vi "AlliGator FLI Dataset Series Actions.vi"(0 "AlliGator Q Elements":T6[](array[typedef]), 1 "VI in":refnum<vi>, 2 "Script in":bool, 5 "AlliGator IV DVR in":refnum<data-value>, 7 "AlliGator Q Event in":T7=enum."GUI:Idle", 9 "Data":variant, 11 "error in (no error)":errorcluster, 12 "AlliGator Ctrl Refnums":T8) -> (3 "Script out":bool, 4 "Alligator Queue Elements":T6[](array[typedef]), 6 "AlliGator IV DVR out":refnum<data-value>, 10 "[Notebook Message]":T1[](array[typedef]) {"Message Style"."Font Size" min=6.0 step=1.0}, 15 "error out":errorcluster)   [LabVIEW 2021, in "AlliGator Action Engine.lvlib"]
doc: "Processes AlliGator FLI Dataset Series-related actions."
uses:
  AlliGator Action Engine.lvlib
  Internal Variables/AlliGator Internal Variables v2.ctl
  <vilib>/vision/Image Controls.llb/IMAQ Image.ctl
  Internal Variables/AlliGator Gate Image Set.ctl
  Files/AlliGator FLI Dataset Type.ctl
  Files/AlliGator Data Series Type.ctl
  Dual-Channel Datasets/AlliGator Dataset Channel.ctl
  Settings/AlliGator Gate Arithmetic.ctl
  Source Image/AlliGator Displayed Image.ctl
  Image/Named ROI Description.ctl
  Phasor Graph/AlliGator Decay Metadata v3.ctl
  Decay Analysis/Decay Preprocessing/AlliGator Decay Background Subtraction Info.ctl
  Decay Analysis/Decay Preprocessing/AlliGator Baseline Subtraction Method.ctl
  Graphs/XY Graph/XY Graph Plot Shift Parameters.ctl
  Graphs/XY Graph/XY Graph Plot Shift Method.ctl
  Decay Analysis/Decay Preprocessing/AlliGator Decay Extrapolation Parameters.ctl
  Phasor/Calibration Phasor (m, phi).ctl
  Phasor/Phasor Reference Series.ctl
  Phasor/Phasor Calibration Map v2.ctl
  Phasor/Phasor (g, s).ctl
  Phasor Graph/AlliGator Raw Phasor Plot Data v5.ctl
  Phasor/Phasor Standard Deviation Options.ctl
  Phasor Plot/AlliGator Phasor Multi-Harmonic Data.ctl
  Phasor/Phasor Harmonic Data.ctl
  Decay Fit Parameter Map/AlliGator Decay Fit Options & Parameters v4.ctl
  Fits/IRF(X)PSED/Decay Fit Options v4.ctl
  Fits/Decay Convolution/Decay Model.ctl
  Fits/Residual Type.ctl
  Fits/IRF(X)PSED/Fit Weights Type v2.ctl
  Fits/Non-linear Fitting Method v2.ctl
  Fits/Fit Calculation Method.ctl
  Fits/Non-linear Fitting Algorithm.ctl
  Decay Analysis/Decay Fit/AlliGator Decay Fit Parameter Constraints 2.ctl
  Fits/IRF(X)PSED/Decay Fit Parameters In List.ctl
  Fits/IRF(X)PSED/MLE Baseline Offset Type.ctl
  Decay Analysis/Decay Preprocessing/AlliGator Decay Preprocessing Parameters.ctl
  Fits/IRF(X)PSED/Decay Fit Parameters & Derived Quantities List v2.ctl
  Fits/IRF(X)PSED/Decay Fit Result Constraint.ctl
  Decay Fit Parameter Map/AlliGator Parameter Maps Data.ctl
  AlliGator Q Event.ctl
  GUI/AlliGator Ctrl Refnums.ctl
  GUI/AlliGator Other Ctrl Refnums.ctl
  GUI/AlliGator State Indicator.ctl
  GUI/AlliGator Main Window Tabs.ctl
  GUI/AlliGator Phasor Plot Ctrl Refnums.ctl
  GUI/AlliGator Phasor Graph Ctrl Refnums.ctl
  Phasor/Phasor Calibration Type.ctl
  GUI/AlliGator Dataset Ctrl Refnums.ctl
  GUI/AlliGator Registered Events Ctrl Refnums.ctl
  GUI/AlliGator Image Histogram Control Refnums.ctl
  Histograms/Linear Histogram Options.ctl
  Histograms/Histogram Bin Option.ctl
  Histograms/Histogram Bin Position.ctl
  Decay Fit Parameter Map/AlliGator Decay Fit Map Control Refnums.ctl
  Parameter Map/AlliGator Parameter Map Control Refnums.ctl
  AlliGator Q Element.ctl
  Notebook/Notebook Message Object.ctl
  Rich Text Box/Text Formatting.ctl
  Rich Text Box/Text Colors.ctl
  Rich Text Box/Text Style.ctl
  Rich Text Box/Text Alignment.ctl
  Rich Text Box/Text Format List.ctl
  Alligator Elements Order in Action Stack.ctl
  Globals, Variables, Constants/AlliGator Variables List.ctl
  Scripts/AlliGator Series Analysis Type.ctl
  Globals, Variables, Constants/AlliGator Globals.vi
  Variant/Variant to Data/Variant to DBL.vi
  Variant/Variant to Data/Variant to Boolean.vi
  AlliGator Add Action Array to Stack.vi
  GUI/GUI.lvlib
  Accumulated Dataset/AlliGator Accumulated Dataset.lvlib
  Scripts/AlliGator Scripts.lvlib
  Sound/Sound.lvlib
  Decay Analysis/Decay Fit/AlliGator Decay Fit.lvlib
  Internal Variables/AlliGator Internal Variables.lvlib
  Image/Image.lvlib
  Variant/Variant to Data/Variant to Data.lvlib
  Source Image/AlliGator Source Image.lvlib
  Globals, Variables, Constants/AlliGator Globals, Variables & Constants.lvlib
  Notebook/Notebook.lvlib
  Phasor/Phasor.lvlib
  Decay Analysis/Decay Preprocessing/AlliGator Decay Preprocessing.lvlib
  Graphs/XY Graph/XY Graph Add-Ons.lvlib
  Phasor Graph/AlliGator Phasor Graph.lvlib
  Files/AlliGator Files.lvlib
  Phasor Plot/AlliGator Phasor Plot.lvlib
  Fits/Fits.lvlib
  Settings/AlliGator Settings.lvlib
  GUI/AlliGator GUI.lvlib
  Decay Fit Parameter Map/AlliGator Decay Fit Parameter Map.lvlib
  Rich Text Box/Rich Text Box.lvlib
  Dual-Channel Datasets/AlliGator Dual-Channel Datasets.lvlib
  Histograms/Histogram Window.lvlib
  Parameter Map/AlliGator Parameter Map.lvlib
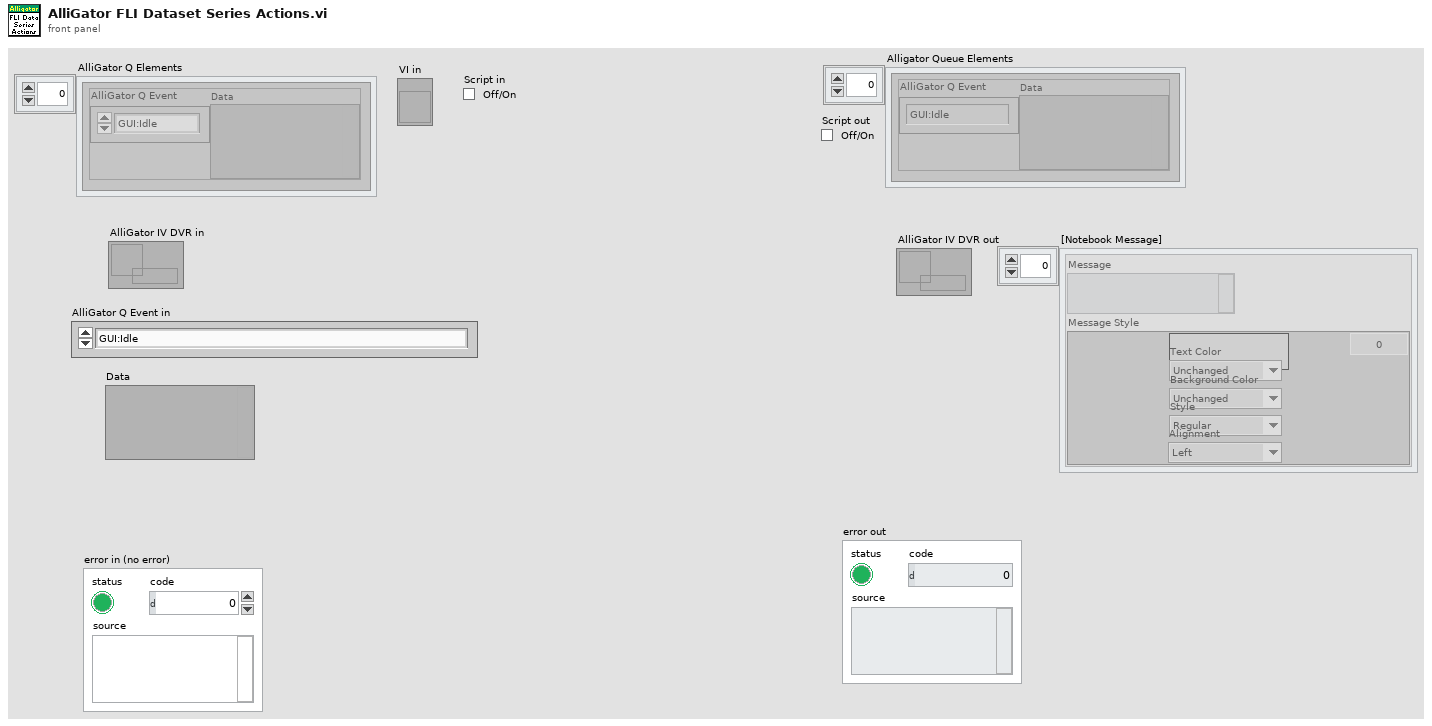
[diagram p1: front panel]
types:
  T1 = typedef "Notebook.lvlib/Notebook Message Object.ctl" = cluster{"Message":string, "Message Style":T2}
  T2 = typedef "Rich Text Box.lvlib/Text Formatting.ctl" = cluster{"Font":string, "Text Color":T3, "Background Color":T3, "Style":T4, "Font Size":dbl, "Alignment":T5}
  T3 = typedef "Rich Text Box.lvlib/Text Colors.ctl" = enum16{"Unchanged", "Black", "Blue", "Cyan", "Maroon", "Gray", "Violet", "Green", "Light Green", "Orange", "Yellow", "Magenta", "Red", "White"}
  T4 = typedef "Rich Text Box.lvlib/Text Style.ctl" = enum16{"Regular", "Bold", "Italic", "Underline", "Strikeout"}
  T5 = typedef "Rich Text Box.lvlib/Text Alignment.ctl" = enum16{"Left", "Right", "Center"}
  T6 = typedef "AlliGator Action Engine.lvlib/AlliGator Q Element.ctl" = cluster{"AlliGator Q Event":T7, "Data":variant}
  T7 = typedef "AlliGator Action Engine.lvlib/AlliGator Q Event.ctl" = enum16{"---- Files ----", "Files:Set Batch Export Files To Save", "Files:Set Dataset Loading & Pre-processing Options", "Files:Check #Frames in Dataset", "Files:Increment Frame Index", "Files:Open Mask Image", "Files:Open White Light Image", "Files:Open Single Dataset", "Files:New Folder of Folders Selected", "Files:Load File (all Types)_Scriptable", "Files:Move Flattened Series to Folders Series", "Files:Select Folder", "Files:Load FLI Dataset", "Files:Load Swiss SPAD 1 Dataset", "Files:Load Swiss SPAD 2 Dataset", "Files:Load .sdt FLI Dataset", "Files:Load .ptu FLI Dataset", "Files:Load .bin FLI Dataset", "Files:Load Single Gate Image Folder", "Files:Load I/m/phi Dataset (deprecated)", "Files:Load Single Image", "Files:Subtract Background File", "Files:Export FLI Dataset", "Files:Load HDF5 FLI Dataset", "Files:Set Destination File Path", "Files:Save Mask Image", "Files:Batch Conversion", "Files:New Folder Selected", "Files:Close FLI Dataset", "Files:Close FLI Dataset Series", "Files:Close White Light Image", "Files:Close Mask Image", "---- FLI Dataset ----", "FLI Dataset:Channel Arithmetic", "FLI Dataset:Export Average Lifetime Map as ASCII", "FLI Dataset:Export User-Defined Quantity Map as ASCII", "FLI Dataset:Python Function FLI Dataset Event", "FLI Dataset:ROI Analysis", "FLI Dataset:Tilted Logistic Square Gated IRF Characteristics Map", "FLI Dataset:Logistic Square Gated IRF Characteristics Map", "FLI Dataset:Square Gated IRF Characteristics Map", "FLI Dataset:Multi-ROI Single-Pixel Phasor Analysis", "FLI Dataset:Multi-ROI Single-Pixel NLSF Analysis", "FLI Dataset:All ROIs IRF Extraction", "FLI Dataset:All ROIs Decay Fit Non-Interactive (Fast + Individual IRF)", "FLI Dataset:All ROIs Phasor Analysis", "FLI Dataset:All ROIs Decay Fit", "FLI Dataset:Fluorescence Decay Statistics", "FLI Dataset:Update Decay Statistics Graph", "FLI Dataset:Get Decay from ROI", "FLI Dataset:All ROIs Average Lifetimes", "FLI Dataset:Save/Load Local IRFs", "FLI Dataset:Clear Local IRFs", "FLI Dataset:Phasor Calibration Maps (# Gates Series) Script", "FLI Dataset:Calibrated Phasor Map Series", "---- FLI Dataset Series ----", "FLI Dataset Series:Sum All Datasets in Series", "FLI Dataset Series:Add Dataset to Accumulated Dataset", "FLI Dataset Series:Display Accumulated Dataset", "FLI Dataset Series:Clear Dataset Series Sum", "FLI Dataset Series:Time-Series Analysis (NLSF)", "FLI Dataset Series:Time-Series Analysis (Phasor)", "---- Image ----", "Image:Update Image Profile Plots", "Image:Image Histogram Cursor Move", "Image:Image Histogram", "Image:Image Contrast", "Image:Set Image Histogram Cursor Move Flag", "Image:Clear Image Overlay", "Image:Use ROI as Search Area", "Image:Set ROI Diameter", "Image:Save Image Data as TIFF", "Image:Save Displayed Image with Overlay", "Image:Save Image Overlay Only", "Image:Save Image as Hot Pixel Mask", "Image:Change Source Image Color Palette", "Image:Copy Image to Clipboard", "Image:Source Image ROI Selection", "Image:Delete All ROIs", "Image:Delete All Unselected ROIs", "Image:Delete ROI", "Image:Merge All ROIs", "Image:Store ROI", "Image:Source Image ROI Storage", "Image:Export ROI Description to Notebook", "Image:Save ROI", "Image:Load ROI", "Image:Paste ROI Definition", "Image:Clear ROI", "Image:Identify ROIs in Mask Image", "Image:Create Complementary ROI", "Image:Create Contour ROI", "Image:Create ROI(s) from Pixels with Peak above Min_Scriptable", "Image:Create ROI(s) from Pixels with Intensity above Min_Scriptable", "Image:Compute ROI Statistics", "Image:Delete ROI(s) based on ROI Characteristics", "Image:Create ROI Grid", "Image:ROI to Individual Pixel ROIs", "Image:Python Function Source Image Event", "Image:Show Phasor Calibration Map ROI Centers", "Image:Convert ROI to Mask Image", "Image:Mouse Move", "Image:Mouse Up", "Image:Set Source Image Mouse Move Flag", "Image:Add Scale Bar Overlay", "Image:Delete Existing ROIs Option", "Image:Overlay ROI Median", "Image:Check Current ROI", "Image:Update True Pixel Value", "---- Decay ----", "Decay:Clear IRF/Reference Plot", "Decay:Add Decay to Graph", "Decay:Smoothen Plot", "Decay:Smoothen Plot Tail", "Decay:Average Selected Plots", "Decay:Extract IRF", "Decay:Optimal IRF Extraction", "Decay:Threshold IRF", "Decay:Fit to Model IRF", "Decay:Fit IRF to Square Gate", "Decay:Fit IRF to Logistic Square Gate", "Decay:Fit IRF to Tilted Logistic Square Gate", "Decay:Create Bounding Cursors Set", "Decay:Export Bounding Cursors Definition to Notebook", "Decay:Denoise Plot", "Decay:Compute Cumulative Function", "Decay:Use as Reference Decay", "Decay:Show Reference Decay/IRF", "Decay:Extrapolate Decay", "Decay:Create Head & Tail Bounding Cursors", "Decay:Store Cursor-defined Head & Tail Fractions", "Decay:Rebin Plot", "Decay:1-Normalize Decay", "Decay:[0-1]-Normalize Plot", "Decay:Straighten Decay", "Decay:Shift Decay", "Decay:Fold Decay", "Decay:Fit Decay", "Decay:Global Fit of Selected Decays", "Decay:Post Global Fit Script", "Decay:Add Global Fit Parameters to Graph", "Decay:Add Decay Parameter(s) to Plot (Graph)", "Decay:Export Decay to Phasor Graph", "Decay:Compute Average Lifetime", "Decay:Plot Convolution", "Decay:Graph Tip Strip Update", "---- Decay Statistics ----", "Decay Statistics:Tip Strip Update", "---- Intensity Time Trace ----", "Intensity Time Trace:Use File Timestamp", "Intensity Time Trace:Load Intensity Corrections File", "Intensity Time Trace:Clear Intensity Corrections File", "Intensity Time Trace:Tip Strip Update", "---- Phasor Plot ----", "Phasor Plot:Build Phasor Plot", "Phasor Plot:Change Phasor Plot Color Palette", "Phasor Plot:Adjust Phasor Plot Display Range", "Phasor Plot:Highlight Image ROI in Phasor Plot", "Phasor Plot:Save Phasor Plot Image with Overlay", "Phasor Plot:Export Complex Phasor Map", "Phasor Plot:Export Phasor Ratio Map", "Phasor Plot:Export Average Lifetime Map", "Phasor Plot:Compute Phase Lifetime Histogram", "Phasor Plot:Compute Phasor Ratio Histogram", "Phasor Plot:Compute Phase Lifetime vs Intensity Scatter Plot", "Phasor Plot:Weber 2-Component Decomposition", "Phasor Plot:Update Phasor Color Map Vertices", "Phasor Plot:Clear Phasor Overlay", "Phasor Plot:Use Segment Extremities as References", "Phasor Plot:Use UC/Segment Intersections as References", "Phasor Plot:Use UC/Principal Axis Intersections as References", "Phasor Plot:Use UC/Linear Fit Intersections as References", "Phasor Plot:Update Phasor Plot Reference", "Phasor Plot:Show Local Phasor Info in Phasor Plot", "Phasor Plot:Update Phasor Plot State", "Phasor Plot:Phasor Plot ROI Storage", "Phasor Plot:Phasor Plot ROI Selection", "Phasor Plot:Python Function Phasor Plot Event", "Phasor Plot:Overlay Phasor ROI, Ratio or Map in Source Image", "Phasor Plot:Compute Decay of Selected Phasors", "Phasor Plot:Phasor at Image Pixel", "Phasor Plot:Mouse Move", "Phasor Plot:Mouse Up", "Phasor Plot:Display Range Mouse Move", "Phasor Plot:Set Mouse Move Flag", "Phasor Plot:Update True Phasor Plot Value", "---- Phasor Graph ----", "Phasor Graph:Get Phasor Value", "Phasor Graph:Create New Phasor Plot Dialog", "Phasor Graph:Update Last Phasor Value", "Phasor Graph:Update Phasor (m, phi)", "Phasor Graph:Remove Single Phasor from Plot", "Phasor Graph:Add Single Phasor to Plot", "Phasor Graph:Remove Phasor Plot", "Phasor Graph:Remove Selected Phasor Plots", "Phasor Graph:Clear Phasor Data", "Phasor Graph:Clear Phasor Graph", "Phasor Graph:Cursor Move", "Phasor Graph:Draw Cursor Connecting Line", "Phasor Graph:Clear Cursor Connecting Line", "Phasor Graph:Find UC Intersection", "Phasor Graph:Use UC/Cursor-Defined Line Intersections", "Phasor Graph:Use Selected Plots Fitted Line/UC Intersections", "Phasor Graph:Use Selected Plots Principal Axis/UC Intersections", "Phasor Graph:Show Single Phasor", "Phasor Graph:Save Single Phasor Plot", "Phasor Graph:Save All Phasor Plots", "Phasor Graph:Load Phasor Plot(s)", "Phasor Graph:Phasor Multiplication", "Phasor Graph:Compute Average Phasor", "Phasor Graph:Compute Multiple Average Phasors (Selected Plots)", "Phasor Graph:Export Single Phasor Plot Phase Lifetimes", "Phasor Graph:Parameter 2 vs Parameter 1 Scatter Plot", "Phasor Graph:Use Cursor n Location", "Phasor Graph:Set Reference n to Current Phase Lifetime Value", "Phasor Graph:Set Reference n to Lifetime Value", "Phasor Graph:Set Cursor n Location", "Phasor Graph:Save Phasor Graph Image", "Phasor Graph:Update SEPL Plot", "Phasor Graph:Export Single Phasor Plot Data", "Phasor Graph:Export Selected Phasor Plots Data", "Phasor Graph:Python Function Phasor Graph Event", "Phasor Graph:Tip Strip Update", "---- Calibration ----", "Calibration:Set Calibration Type", "Calibration:Load/Save Phasor Calibration", "Calibration:Load/Save Phasor Calibration Series", "Calibration:Load/Save Phasor Calibration Map", "Calibration:Use as Calibration", "Calibration:Compute Optimal Calibration from Phasor References", "Calibration:Clear Phasor Calibration", "Calibration:Single Phasor Calibration Information", "Calibration:Use as Calibration Series", "Calibration:Use as Calibration Map", "Calibration:Clear Calibration Series", "Calibration:Phasor Calibration Series Information", "Calibration:Clear Calibration Map", "Calibration:Phasor Calibration Map Information", "Calibration:Apply Phasor Calibration", "Calibration:Update Single Plot Calibration", "Calibration:Update Multiple Plots Calibration", "Calibration:Clear Single Plot Calibration", "Calibration:Clear All Plots Calibrations", "Calibration:Clear Plot(s) Calibration(s)?", "---- Phasor Ratio ----", "Phasor Ratio:Clear Reference n", "Phasor Ratio:Toggle Selected Plot(s)  Lock to Reference 1", "Phasor Ratio:Use as Reference n", "Phasor Ratio:Send Reference n to Notebook", "Phasor Ratio:Toggle Selected Plot(s)  Lock to Reference 2", "Phasor Ratio:Compute Phasor Ratio at Mouse Location", "Phasor Ratio:Compute Phasor Plot's Average Phasor Ratio", "Phasor Ratio:Compute Time-Series Phasor Ratios", "Phasor Ratio:Fit Line to Phasor Ratio Plot", "Phasor Ratio:Save References", "Phasor Ratio:Load References", "Phasor Ratio:Update Phasor Reference 1", "Phasor Ratio:Update Phasor Reference 2", "Phasor Ratio:Move Cursor n to Reference n", "Phasor Ratio:Use as Phasor Reference 1 Lifetime", "Phasor Ratio:Use as Phasor Reference 2 Lifetime", "Phasor Ratio:Export Phasor Ratio Map as ASCII", "Phasor Ratio:Tip Strip Update", "---- Lifetime & Other Parameters Graph ----", "Lifetime:Compute Sliced Mean, SDV and CV Plots", "Lifetime:Plot Decay Shifts", "Lifetime:Plot Histogram", "---- Decay Fit Parameter Map ----", "Decay Fit Parameter Map:Export ROI NLSF Data as ASCII", "Decay Fit Parameter Map:Set Decay Fit Parameter Map Selection", "Decay Fit Parameter Map:Build Decay Fit Parameter Map", "Decay Fit Parameter Map:Change Decay Fit Parameter Map Color Palette", "Decay Fit Parameter Map:Export Decay Fit Parameter Map Data as ASCII", "Decay Fit Parameter Map:Export All Decay Fit Parameter Maps Data as ASCII", "Decay Fit Parameter Map:Selected Parameter Scatterplot", "Decay Fit Parameter Map:Parameter 2 vs Parameter 1 Scatterplot", "Decay Fit Parameter Map:Save Decay Fit Parameter Map Image", "Decay Fit Parameter Map:Save-Load IRFs & Fit Data", "Decay Fit Parameter Map:Update Local Decay Plots", "Decay Fit Parameter Map:Python Function Decay Fit Parameters Map Event", "Decay Fit Parameter Map:Overlay Decay Fit Parameter Map in Source Image", "Decay Fit Parameter Map:Selected Parameter vs Intensity Scatterplot", "Decay Fit Parameter Map:Mouse Up", "Decay Fit Parameter Map:Mouse Move", "Decay Fit Parameter Map:Display Range Mouse Move", "Decay Fit Parameter Map:Change Map Resolution", "Decay Fit Parameter Map:Variance Significance Maps", "Decay Fit Parameter Map:Fit Result Constraints Window", "---- Parameter Map ----", "Parameter Map:Export ROI Parameters Data as ASCII", "Parameter Map:Add Parameter Map Set", "Parameter Map:Delete Parameter Map Set", "Parameter Map:Update Parameter List", "Parameter Map:Build Parameter Map", "Parameter Map:Change Parameter Map Color Palette", "Parameter Map:Export Parameter Map Data as ASCII", "Parameter Map:Export All Parameter Maps Data as ASCII", "Parameter Map:Selected Parameter Scatterplot", "Parameter Map:Parameter 2 vs Parameter 1 Scatterplot", "Parameter Map:Selected Parameter vs Intensity Scatterplot", "Parameter Map:Save Parameter Map Image", "Parameter Map:Save-Load IRFs & Parameter Maps (TODO)", "Parameter Map:Set Parameter Map Selection", "Parameter Map:Python Function Parameter Map Event", "Parameter Map:Overlay Parameter Map in Source Image", "Parameter Map:Update Local Decay Plots", "Parameter Map:Mouse Up", "Parameter Map:Mouse Move", "Parameter Map:Display Range Mouse Move", "---- Generic Graph ----", "Generic Graph:Generic XY Graph Event", "Generic Graph:Python Function XY Graph Event", "Generic Graph:New Plot", "Generic Graph:Save Plot", "Generic Graph:XY Plot Histogram", "Generic Graph:Set XY Graph Plot Name", "Generic Graph:Set Last Cursor Style", "Generic Graph:Tip Strip Update", "---- GUI ----", "GUI:Start Script", "GUI:Type of Displayed Image Changed", "GUI:Gate Image Slide Changed", "GUI:Show Busy Icon", "GUI:Show Busy Icon & Abort Button", "GUI:Hide Busy Icon", "GUI:Hide Busy Icon & Abort Button", "GUI:Abort", "GUI:End Script", "GUI:Start Timing", "GUI:End Timing", "GUI:Set State Indicator", "GUI:Send Parameters JSON Strings to Clipboard", "GUI:Set Gate Step", "GUI:Idle", "GUI:Initialization", "GUI:Quit", "GUI:Increment Dataset Index", "GUI:Set Dataset Index to -1", "GUI:Time Series Slider Moved", "GUI:Time Series Slider Changed", "GUI:Toggle Playback or Loop", "GUI:Playback Script", "GUI:Set Phasor Frequency", "GUI:Open Window", "GUI:Start Test Script", "GUI:End Test Script", "GUI:Set Verbose Mode", "GUI:Set Verbose Settings Mode", "DEBUG"}
  T8 = typedef "AlliGator GUI.lvlib/AlliGator Ctrl Refnums.ctl" = cluster{"Other AlliGator Ctrl Refnums":T9, "Phasor Plot Ctrl Refnums":T10, "Phasor Graph Ctrl Refnums":T11, "Dataset Control Refnums":T12, "Registered Events Ctrl Refnums":T13, "Image Histogram Ctrl Refnums":T14, "Decay Fit Map Ctrl Refnums":T15, "Parameter Map Ctrl Refnums":T16}
  T9 = typedef "AlliGator GUI.lvlib/AlliGator Other Ctrl Refnums.ctl" = cluster{"State Indicators":refnum<vi>, " Progress Bar":refnum<vi>, "Decay Graph Active":refnum<vi>, "Decay Statistics Bin":refnum<vi>, "Time Step":refnum<vi>, "Use File Timestamp":refnum<vi>, "Tab Control":refnum<vi>, "CPU":refnum<vi>, "Abort Fit":refnum<vi>, "Dataset File/Folder Path":refnum<vi>, "Abort ROI Creation":refnum<vi>, "Event LED":refnum<vi>, "Dataset File/Folder Path 2":refnum<vi>, "Dataset File/Folder Path 3":refnum<vi>, "Dataset File/Folder Path 4":refnum<vi>, "Dataset File/Folder Path 5":refnum<vi>, "Dataset File/Folder Path 6":refnum<vi>, "Dataset File/Folder Path 7":refnum<vi>, "Dataset File/Folder Path 8":refnum<vi>, "Dataset File/Folder Path 9":refnum<vi>, "Dataset File/Folder Path 10":refnum<vi>, "Dataset File/Folder Path 11":refnum<vi>}
  T10 = typedef "AlliGator GUI.lvlib/AlliGator Phasor Plot Ctrl Refnums.ctl" = cluster{"Phasor Ratio":refnum<vi>, "Modulus Lifetime":refnum<vi>, "Phasor at cursor (m, phi)":refnum<vi>, "Phase Lifetime":refnum<vi>, "Phasor at cursor (g, s)":refnum<vi>, "Phasor Plor Average Lifetime":refnum<vi>, "Phasor Plot Active":refnum<vi>, "Save Phasor Plot":refnum<vi>, "Image Overlay Color":refnum<vi>, "Phasor Plot Color Scale":refnum<vi>, "Reference 1 Button":refnum<vi>, "Reference 2 Button":refnum<vi>, "True Phasor Plot Value":refnum<vi>}
  T11 = typedef "AlliGator GUI.lvlib/AlliGator Phasor Graph Ctrl Refnums.ctl" = cluster{"Phasor Ratio":refnum<vi>, "Modulus Lifetime":refnum<vi>, "Phasor at cursor (m, phi)":refnum<vi>, "Phase Lifetime":refnum<vi>, "Phasor at cursor (g, s)":refnum<vi>, "Phasor Graph Average Lifetime":refnum<vi>, "Phasor Graph Active":refnum<vi>, "Save Phasor Graph":refnum<vi>, "Phasor Frame Slide":refnum<vi>, "Single Step Phasor":refnum<vi>, "Calibration Type":refnum<vi>, "Show Line":refnum<vi>, "Phase Lifetime 1":refnum<vi>, "Phase Lifetime 2":refnum<vi>, "Phasor Graph Frequency":refnum<vi>, "Phasor Reference 1 Control":refnum<vi>, "Phasor Reference 2 Control":refnum<vi>, "Calibration Lifetime":refnum<vi>, "Phase Lifetime SDV":refnum<vi>, "Average Lifetime SDV":refnum<vi>, "Phasor Ratio SDV":refnum<vi>, "Modulus Lifetime SDV":refnum<vi>}
  T12 = typedef "AlliGator GUI.lvlib/AlliGator Dataset Ctrl Refnums.ctl" = cluster{"Current Data":refnum<vi>, "Gate Image Slide":refnum<vi>, "Time Point Slide":refnum<vi>, "Current Time Stamp":refnum<vi>, "Save Image":refnum<vi>, "Displayed Image":refnum<vi>, "Overlay Mode":refnum<vi>, "Phasor Overlay Color":refnum<vi>, "Image Color Scale":refnum<vi>, "Use ROI as Search Area":refnum<vi>, "Source Image ROI Color":refnum<vi>, "True Pixel Value":refnum<vi>}
  T13 = typedef "AlliGator GUI.lvlib/AlliGator Registered Events Ctrl Refnums.ctl" = cluster{"Time Point Slider":refnum<vi>, "Phasor Plot Display Range":refnum<vi>, "Decay Graph":refnum<vi>, "Decay Statistics Graph":refnum<vi>, "Intensity Time Trace":refnum<vi>, "Phasor Graph":refnum<vi>, "Phasor Ratio Graph":refnum<vi>, "Lifetime Graph":refnum<vi>, "Phasor Plot Display":refnum<vi>, "Source Image Display":refnum<vi>, "Decay Fit Parameter Map Display Range":refnum<vi>, "Decay Fit Parameter Map Display":refnum<vi>, "Parameter Map Display Range":refnum<vi>, "Parameter Map Display":refnum<vi>, "Phasor Plot Display Range":refnum<vi>}
  T14 = typedef "AlliGator GUI.lvlib/AlliGator Image Histogram Control Refnums.ctl" = cluster{"Image Histogram":refnum<vi>, "Image Histogram Options":refnum<vi>, "Image Histogram Active":refnum<vi>, "Image Histogram Upper Percentile":refnum<vi>, "Image Histogram Lower Percentile":refnum<vi>, "Auto-Adjust Contrast":refnum<vi>}
  T15 = typedef "AlliGator Decay Fit Parameter Map.lvlib/AlliGator Decay Fit Map Control Refnums.ctl" = cluster{"Decay Fit Parameter Map Color Scale":refnum<vi>, "Decay Fit Parameter":refnum<vi>, "Max Parameter":refnum<vi>, "Min Parameter":refnum<vi>, "Decay Fit Parameter Map Display":refnum<vi>, "Decay Fit Parameter Map Display Range":refnum<vi>, "Decay Parameter Map X":refnum<vi>, "Decay Parameter Map Y":refnum<vi>, "Decay Parameter Map Value":refnum<vi>}
  T16 = typedef "AlliGator Parameter Map.lvlib/AlliGator Parameter Map Control Refnums.ctl" = cluster{"Parameter Map Color Scale":refnum<vi>, "Map Parameter":refnum<vi>, "Max Parameter":refnum<vi>, "Min Parameter":refnum<vi>, "Parameter Map Display":refnum<vi>, "Parameter Map Display Range":refnum<vi>, "Parameter Map Set":refnum<vi>, "Parameter Map X":refnum<vi>, "Parameter Map Y":refnum<vi>, "Parameter Map Value":refnum<vi>}
  T17 = typedef "Notebook.lvlib/Text Format List.ctl" = enum16{"Message", "Result", "Error", "Setting", "Verbose", "Warning"}
  T18 = typedef "AlliGator Globals, Variables & Constants.lvlib/AlliGator Variables List.ctl" = enum16{"---- GUI ----", "GUI:Initialization Status", "GUI:State Indicators Refnum", "GUI:Original AlliGator Menu Items", "GUI:Current Action Loop State", "GUI:Script in progress", "GUI:Playback", "GUI:Loop Playback", "GUI:Search ROI Used", "GUI:Search ROI", "Decay Graph Max Legend Size", "Intensity Graph Max Legend Size", "Decay Statistics Graph Max Legend Size", "Phasor Graph Max Legend Size", "Phasor Ratio Graph Max Legend Size", "Lifetime Graph Max Legend Size", "---- Files ----", "Files:Export Dataset Frames as Individual Files", "Files:Show Batch Export Help Balloons", "Files:Frames in Dataset", "Files:ptu File Frame Start Indices", "Files:Current Frame in Dataset", "Files:Current Frame Timestamp", "Files:Dataset Loaded", "Files:Dataset Metadata", "Files:Dataset Channel", "Files:Dataset Data Description", "Files:Background Dataset Metadata", "Files:Background Dataset Channel", "Files:Background Dataset Data Description", "Files:Background File Subtraction", "Files:Background File Path", "Files:Background File Pile-up Correction", "Files:Background File Pixel Well Capacity", "Files:Background File Scaling Factor", "Files:Current Dataset Load Settings", "Files:Dataset Path", "Files:ICCD-specific Information", "Files:Macrotime Gate Separation", "------ Python Plugins ------", "Python Plugins:Information", "Python Plugins:Python Session", "Python Plugins:Valid Python Session?", "---- Source Image ----", "Source Image:ROIs", "Source Image:Current ROI", "Source Image:ROI Event Refnum", "X_Source Image:Display Range", "X_Source Image:Palette Information", "X_Source Image:Type of Displayed Image", "X_Time Gate Slider", "Source Image:Palette List", "Source Image:Scale", "Source Image:ROI Overlay Color", "Source Image:Overlay to Erase", "Source Image:Is Displayed Image Accumulated", "Source Image:White Light Image Modified", "Source Image:Mask Image Modified", "---- Image Profile Window ----", "Image Profile:Window Event Refnum", "Image Profile:IntensityType", "Image Profile:Intensity Average Type", "Image Profile:Intensity-weighted SDV", "Image Profile:Box Profile Type", "Image Profile:Window Open", "Image Profile:Plotted Fit Parameter", "------ Phasor Graph -------", "Phasor Graph:Show Line", "---- Phasor Plot ---", "Phasor Plot:Parameters Changed", "Phasor Plot:FLI Dataset Modified since last Calculation", "Phasor Harmonics Data", "Selected Phasor Harmonics", "Phasor Harmonic Manager Event Refnum", "Phasor Plot:ROIs", "Phasor Plot:Current ROI", "Phasor Plot:ROI Event Refnum", "Phasor Plot:Image Reference Points", "Phasor Plot:Computed", "Phasor Plot:Palette Information", "Phasor Plot:Palette List", "Phasor Plot:Phasor Ratio Palette Information", "Phasor Plot:Phasor Ratio Palette List", "Phasor Plot:Image Scale", "Phasor Plot:Image Overlay to Erase", "Phasor Plot:Image Elements to Update", "Phasor Plot:Current Calculation Parameters", "Phasor Plot:Current Calibration Options", "Phasor Plot:Reset Cumulated Phasor Plot", "Phasor Plot:Reference 1", "Phasor Plot:Lifetime Reference 1", "Phasor Plot:Reference 1 Frequency", "Phasor Plot:Reference 2", "Phasor Plot:Lifetime Reference 2", "Phasor Plot:Reference 2 Frequency", "---- Decay Analysis ----", "Number of Selected Decays to Fit", "LS Fit Results", "LAR Fit Results", "BS Fit Results", "Last Decay Max - Min", "Best Fit Parameters", "Best Fit Parameter Names", "Actual Size X", "Actual Size Y", "Binning X", "Binning Y", "Actual # Gates", "Dataset Number", "Gates to...", "Gates Skipped", "Gates to keep", "Gate Step", "Gate Separation", "Reversed Gates", "Pile-up Correction", "Pixel Well Capacity", "Background Subtracted", "Background Subtraction Method", "Background Definition Range", "Background File (deprecated)", "Number of Dataset Accumulated", "Array of Accumulated Dataset Paths", "Do Averaged Datasets", "Destination File Path", "Process Plot Target", "Use 1/D as Phasor Frequency", "---- Decay Fit Parameter Map -----", "Decay Fit Parameter Map:Palette Information", "Decay Fit Parameter Map:Palette List", "Decay Fit Parameter Map:X Resolution", "Decay Fit Parameter Map:Y Resolution", "Decay Fit Parameter Map:Use Decay Fit Result Constraints", "Decay Fit Parameter Map:Decay Fit Result Constraints", "Decay Fit Parameter Map:Decay Fit Result Constraints Applied", "---- Parameter Map ----", "Parameter Map:Palette Information", "Parameter Map:Palette List", "------- Local Decay Window ---------", "Local Decay Graph Window:Event Refnum", "Local Decay Graph Window:Use normalized IRF for convolution", "----- Miscellaneous ----", "Misc:Skippable Dialog Windows Status"}
  T19 = typedef "AlliGator Action Engine.lvlib/Alligator Elements Order in Action Stack.ctl" = enum16{"Enqueue 2 AFTER 1", "Enqueue 2 BEFORE 1"}
  T20 = typedef "AlliGator Scripts.lvlib/AlliGator Series Analysis Type.ctl" = enum16{"Current ROI (Fixed)", "All ROIs (Fixed)", "Sequential ROIs"}
  T21 = typedef "AlliGator Internal Variables.lvlib/AlliGator Internal Variables v2.ctl" = cluster{"----------------------------- Images -----------------------------":u8, "Displayed Image":T22, "White Light Image":T22, "Mask Image":T22, "ROI Mask Image":T22, "Current Dataset Images 1":T23, "Background Dataset Images 1":T23, "Current Dataset Images 2":T23, "Background Dataset Images 2":T23, "Current Dataset Arithmetic Images":T23, "Accumulated Dataset Images 1":T23, "Accumulated Dataset Images 2":T23, "Accumulated Dataset Arithmetic Images":T23, "----------------------------- File Paths -----------------------------":u8, "Phasor Plot Image":T22, "Decay Fit Parameter Map Image":T22, "Parameter Map Image":T22, "Single Data Point Path":path, "White Light Image Path":path, "Mask Image Path":path, "Time-Series Folder":path, "[Time-Series Paths]":path[], "----------------------------- FLI Dataset -----------------------------":u8, "Current Dataset":i32, "Single Dataset Type":T24, "Current Folder":string, "AlliGator Data Series Type":T25, "# Datasets":i32, "Dual-Channel Dataset":bool, "Selected Channel Name":string, "Dataset Channel":T26, "Channel Arithmetic":T27, "Dual-Channel Background Dataset":bool, "Background Channel":T26, "Dual-Channel Accumulated Dataset":bool, "Start Time":dbl, "[Time-Series Timestamps]":dbl[], "[Intensity Corrections]":dbl[], "Time Series Script":bool, "Type of Displayed Image":T28, "Gate Image Slide":u16, "# Gates":i32, "ROIs":T29[], "----------------------------- Decays -----------------------------":u8, "ROI Decay":cluster{"t Array":dbl[], "I Array":dbl[]}, "Valid Decay":bool, "Decay  Metadata":T31, "Reference Decay Plot Name":string, "Reference Decay":cluster{"t Array":dbl[], "I Array":dbl[]}, "Decay Shift Plot":cluster{"Time Stamps":dbl[], "Decay Shifts":dbl[]}, "[Decays Max Values]":sgl[], "[Decays Min Values]":sgl[], "----------------------------- Calibration -----------------------------":u8, "Calibration Phasor":T37, "Calibration Phasor Series":T38, "Phasor Calibration Map":T39, "Calibration Map MD5 Digest":string, "----------------------------- Phasor Graph -----------------------------":u8, "Last Raw Phasor":T40, "Last Calibrated Phasor":T40, "Last Calibrated Phasor SDV":T40, "Phasor Graph:Phasor Plot":cluster{"g Array":dbl[], "s Array":dbl[]}, "Phasor Graph:Phasor SDV Plot":cluster{"g Array":dbl[], "s Array":dbl[]}, "[Phasor Graph:Raw Phasor Plots]":T41[], "Phasor Plot locked to Ref 1":i32, "[Phasor Plot(s) locked to Ref 1]":i32[], "[Phasor Plot(s) locked to Ref 2]":i32[], "[Pixel Phasors]":T40[], "----------------------------- Phasor Plot -----------------------------":u8, "[[Sum Image]]":dbl[][], "[[CSG Phasors]]":csg[][], "[[Valid Pixel?]]":bool[][], "[[Phasor Ratios]]":dbl[][], "[[Average Lifetimes]]":dbl[][], "Amplitude Weighted Average Lifetime":bool, "I/m/phi Dataset":cluster{"I/m/phi Dataset?":bool, "Base Frequency":dbl[unit], "Harmonic Orders":u8[]}, "Multi Phasor Plot Data":T43, "----------------------------- Decay Fit Parameter Map -----------------------------":u8, "Decay Fit Options & Parameters":T45, "Fit Options: Decay Preprocessing Parameters":T56, "Fit Options: Reference Decay":cluster{"t Array":dbl[], "I Array":dbl[]}, "Is Full Image Parameters Map":bool, "Is Single-Pixels Parameters Map":bool, "NLSF Parameters Map X Resolution":i32, "NLSF Parameters Map Y Resolution":i32, "[Single Decay Fit Parameters]":dbl[], "Fit Model":T47, "[[Multiple Decays Fit Parameters]]":dbl[][], "[[Multiple Decays Fit Parameter SDVs]]":dbl[][], "[[IRFs]]":dbl[][], "[ROI Descriptors]":T30[], "IRF Array Time Axis":dbl[], "Decay Array Time Axis":dbl[], "[Decay Fit Parameter Names]":T57[], "[Decay Sum]":dbl[], "Array of Decay Fit Result Constraints":T58[], "Selected ROIs Array":bool[], "----------------------------- Parameter Maps -----------------------------":u8, "[Map Set Names]":string[], "[Parameter Maps]":T59[], "[[User-defined Quantities]]":dbl[][], "User-defined Quantity":string}
  T22 = typedef "IMAQ Image.ctl" = refnum<image>
  T23 = typedef "AlliGator Internal Variables.lvlib/AlliGator Gate Image Set.ctl" = cluster{"SGL Gate Images":T22[], "SGL Sum Image":T22, "SGL Max Image":T22, "SGL Min Image":T22}
  T24 = typedef "AlliGator Files.lvlib/AlliGator FLI Dataset Type.ctl" = enum16{"HDF5 FLI Dataset", "Gate Image Folder", ".sdt FLI Dataset (Becker & Hickl)", ".ptu FLI Dataset (PicoQuant)", "SS1 FLI Dataset", "SS2 FLI Dataset", "I/m/phi Dataset", ".bin FLI Dataset (PicoQuant Binned)", ".bin FLI Dataset (Piccolo Binned)", ".mat FLI Dataset"}
  T25 = typedef "AlliGator Files.lvlib/AlliGator Data Series Type.ctl" = enum16{"Not a Supported Series", "Gate Images Folder Series", "SwissSPAD 2 Dataset Series", "B&H FLI Dataset Series", "PicoQuant PTU FLI Dataset Series", "PicoQuant BIN FLI Dataset Series", "Piccolo hist BIN FLI Dataset Series", "HDF5 FLI Dataset Series"}
  T26 = typedef "AlliGator Dual-Channel Datasets.lvlib/AlliGator Dataset Channel.ctl" = enum16{"G2", "INT"}
  T27 = typedef "AlliGator Settings.lvlib/AlliGator Gate Arithmetic.ctl" = enum16{"None", "INT-G2", "G2/INT*<INT>", "(1 - G2/INT)*<INT>"}
  T28 = typedef "AlliGator Source Image.lvlib/AlliGator Displayed Image.ctl" = enum16{"Single Gate", "Sum of All Gates", "Max of All Gates", "Min of All Gates", "-", "White Ligth Image", "Mask Image"}
  T29 = typedef "Image.lvlib/Named ROI Description.ctl" = cluster{"ROI Descriptor":T30, "ROI Name":string, "Overlay Color":u32}
  T30 = typedef "ROI Descriptor" = cluster{"Global Rectangle":i32[], "Contours":cluster{"ID":enum32{"External", "Internal"}, "Type":u32, "Coordinates":i32[]}[]}
  T31 = typedef "AlliGator Phasor Graph.lvlib/AlliGator Decay Metadata v3.ctl" = cluster{"ROI Descriptor":T30, "ROI Center":cluster{"X":i32, "Y":i32}, "Decay Background Subtraction Info":T32, "Decay Reverted":bool, "Decay Smoothened":bool, "Decay Straightened":bool, "Fitted Tau (Decay Straightening)":dbl, "Decay Shift Parameters":T34, "Decay Shifted":bool, "Decay Extrapolated":bool, "Decay Extrapolation Parameters":T36, "Decay Normalized":bool, "Fold Decay":bool, "# Folds":u32}
  T32 = typedef "AlliGator Decay Preprocessing.lvlib/AlliGator Decay Background Subtraction Info.ctl" = cluster{"Laser Period":dbl[unit], "Gate Duration":dbl[unit], "Baseline Subtraction Method":T33, "Background Definition Range":cluster{"Min Gate":dbl[unit], "Max Gate":dbl[unit]}, "Total Intensity w/o Bkgd Subtraction":dbl, "Bkgd-subtracted Intensity (exp)":dbl, "# Data Points":i32, "Background/Gate":dbl, "Fitted Lifetime":dbl[unit], "Bkgd-subtracted Intensity (theo)":dbl}
  T33 = typedef "AlliGator Decay Preprocessing.lvlib/AlliGator Baseline Subtraction Method.ctl" = enum16{"Mean", "Min", "Square Gated Single-Exponential", "File", "Constant"}
  T34 = typedef "XY Graph Add-Ons.lvlib/XY Graph Plot Shift Parameters.ctl" = cluster{"Type":T35, "Shift":dbl[unit], "Threshold":dbl, "Rotate":bool}
  T35 = typedef "XY Graph Add-Ons.lvlib/XY Graph Plot Shift Method.ctl" = enum16{"Default", "CFD", "Threshold", "Cross-Correlation"}
  T36 = typedef "AlliGator Decay Preprocessing.lvlib/AlliGator Decay Extrapolation Parameters.ctl" = cluster{"Additional Points":u32, "Head Fraction":dbl, "Fitted Tau":dbl, "Use Periodicity":bool, "Use Cursors":bool, "Tail Fraction":dbl}
  T37 = typedef "Phasor.lvlib/Calibration Phasor (m, phi).ctl" = cluster{"m":dbl, "phi":dbl, "Phasor Frequency":dbl[unit], "Reference Lifetime":dbl[unit]}
  T38 = typedef "Phasor.lvlib/Phasor Reference Series.ctl" = cluster{"m Array":dbl[], "phi Array":dbl[], "Phasor Frequency":dbl[unit], "Calibration Lifetime":dbl[unit]}
  T39 = typedef "Phasor.lvlib/Phasor Calibration Map v2.ctl" = cluster{"Phasor Frequency":dbl[unit], "Calibration Lifetime":dbl[unit], "ROI Centers":cluster{"X":i32, "Y":i32}[], "ROI Descriptors":T30[], "Map Resolution X":i32, "Map Resolution Y":i32, "z Array":cdb[]}
  T40 = typedef "Phasor.lvlib/Phasor (g, s).ctl" = cluster{"g":dbl, "s":dbl}
  T41 = typedef "AlliGator Phasor Graph.lvlib/AlliGator Raw Phasor Plot Data v5.ctl" = cluster{"Phasor Plot Name":string, "Raw Phasor Plot":T40[], "Phasor Frequency":dbl[unit], "[Decay Metadata]":T31[], "Raw Phasor Plot SDV":T40[], "Phasor SDV Options":T42, "[Calibration Phasor]":T37[], "Intensity Array":dbl[]}
  T42 = typedef "Phasor.lvlib/Phasor Standard Deviation Options.ctl" = cluster{"Compute Estimated SDV":bool, "# Replicas":u32, "Use Estimated Average Phasor":bool}
  T43 = typedef "AlliGator Phasor Plot.lvlib/AlliGator Phasor Multi-Harmonic Data.ctl" = cluster{"Base Frequency":dbl[unit], "# Harmonics":u8, "Harmonic Orders":u8[], "Phasor Plot Settings Checksum":u64, "Phasor Harmonic Data Array":T44[]}
  T44 = typedef "Phasor.lvlib/Phasor Harmonic Data.ctl" = cluster{"Phasor Harmonic Name":string, "Phasor Plot Settings Checksum":u64, "Phasor Frequency":dbl[unit], "Base Frequency":dbl[unit], "Harmonic Order":u8, "Phasor Plot Parameters":string, "Phasor Array [[CSG]]":csg[][], "Dataset File Path":path}
  T45 = typedef "AlliGator Decay Fit Parameter Map.lvlib/AlliGator Decay Fit Options & Parameters v4.ctl" = cluster{"SYNC Period":dbl[unit], "Fit Options":T46, "Fit Parameter Constraints":T53[], "MLE Baseline Offset":dbl, "MLE Baseline Offset Type":T55}
  T46 = typedef "Fits.lvlib/Decay Fit Options v4.ctl" = cluster{"Show Fit Residuals":bool, "Fit Model":T47, "Residual Type":T48, "Max Decay Percentile":dbl, "Min Decay Percentile":dbl, "Show Full Decay":bool, "Weights":T49, "Fitting Method":T50, "Compute Parameter Uncertainties":bool, "Periodic Boundaries":bool, "Model Calculation":T51, "Period":dbl[unit], "Termination Criteria":cluster{"Max Iterations":i32, "Max Function Calls":i32, "Max Time":dbl[unit], "Function Tolerance":dbl, "Parameter Tolerance":dbl, "Gradient Tolerance":dbl, "Min Lambda":dbl, "Max Lambda":dbl, "Initial Tick Count":u32}, "Offset Resolution":dbl[unit], "Use Local IRF":bool, "Fitting Algorithm":T52, "Show Confidence Interval ":bool, "Confidence Level":dbl}
  T47 = typedef "Fits.lvlib/Decay Model.ctl" = enum16{"1-Exponential", "2-Exponentials"}
  T48 = typedef "Fits.lvlib/Residual Type.ctl" = enum16{"Standard", "Normalized", "Reduced"}
  T49 = typedef "Fits.lvlib/Fit Weights Type v2.ctl" = enum16{"Unweighted", "1/Variance (Neyman)", "1/Variance (Pearson)", "Best of All"}
  T50 = typedef "Fits.lvlib/Non-linear Fitting Method v2.ctl" = enum16{"Least Square", "Least Absolute Residual", "Bisquare", "MLE", "-", "Best of All"}
  T51 = typedef "Fits.lvlib/Fit Calculation Method.ctl" = enum16{"Simulation", "Convolution", "Integration"}
  T52 = typedef "Fits.lvlib/Non-linear Fitting Algorithm.ctl" = enum16{"Levenberg-Marquardt", "Trust-Region Dogleg"}
  T53 = typedef "AlliGator Decay Fit.lvlib/AlliGator Decay Fit Parameter Constraints 2.ctl" = cluster{"Fit Parameter":T54, "Min Value":dbl, "Max Value":dbl, "Global":bool, "Used":bool}
  T54 = typedef "Fits.lvlib/Decay Fit Parameters In List.ctl" = enum16{"Offset", "Baseline", "A_1", "tau_1", "A_2", "tau_2"}
  T55 = typedef "Fits.lvlib/MLE Baseline Offset Type.ctl" = enum32{"Absolute", "Percentage"}
  T56 = typedef "AlliGator Decay Preprocessing.lvlib/AlliGator Decay Preprocessing Parameters.ctl" = cluster{"Background Subtraction":bool, "Straighten Decay":bool, "Reverse Gates":bool, "1-Normalized Decay":bool, "Smoothen Decay":bool, "Smoothing Parameter":dbl, "Shift Decay":bool, "Decay Shift Parameters":T34, "Extrapolate Decay":bool, "Additional Points":u32, "Head Fraction":dbl, "Pixel-Normalize Decay":bool, "Use Periodicity":bool, "Use Cursors":bool, "Tail Fraction":dbl, "Use Decay Pre-Processing":bool, "Fold Decay":bool, "# Folds":u32, "[0-1]-Normalized Decay":bool}
  T57 = typedef "Fits.lvlib/Decay Fit Parameters & Derived Quantities List v2.ctl" = enum16{"Offset", "Baseline", "A_1", "tau_1", "A_2", "tau_2", "<tau>_a", "f1_a", "f2_a", "<tau>_i", "f1_i", "f2_i", "-", "R^2", "Chi^2"}
  T58 = typedef "Fits.lvlib/Decay Fit Result Constraint.ctl" = cluster{"Fit Parameter":enum16{"Offset", "Baseline", "A_1", "tau_1", "A_2", "tau_2", "<tau>_a", "f1_a", "f2_a", "<tau>_i", "f1_i", "f2_i", "-", "R^2", "Chi^2", "Max Relative Residual", "<Residual ACF>", "Residual ACF SDV", "tau_2/tau_1"}, "Min Value":dbl, "Max Value":dbl, "Use Constraint":bool}
  T59 = typedef "AlliGator Decay Fit Parameter Map.lvlib/AlliGator Parameter Maps Data.ctl" = cluster{"Map Set Name":string, "[Parameter Names]":string[], "[[Parameters]]":dbl[][], "[[Parameter SDVs]]":dbl[][], "Decay Array Time Axis":dbl[], "[[IRFs]]":dbl[][], "IRF Array Time Axis":dbl[], "X Resolution":i32, "Y Resolution":i32, "Intensity Array":dbl[]}
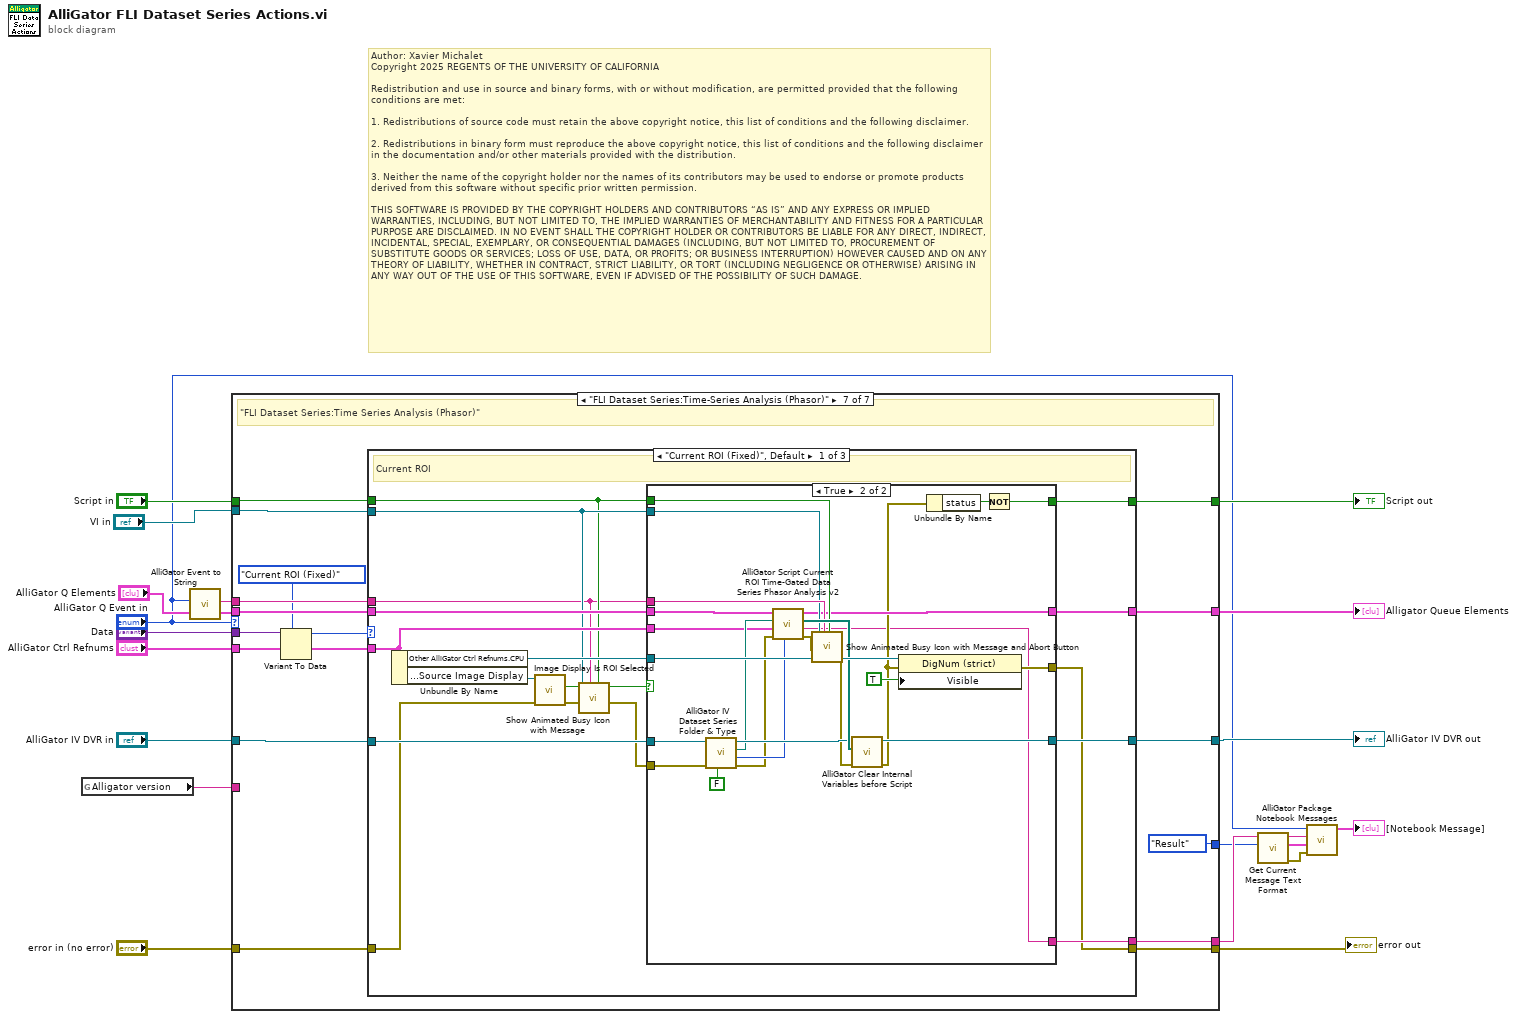
[diagram p0: block diagram]
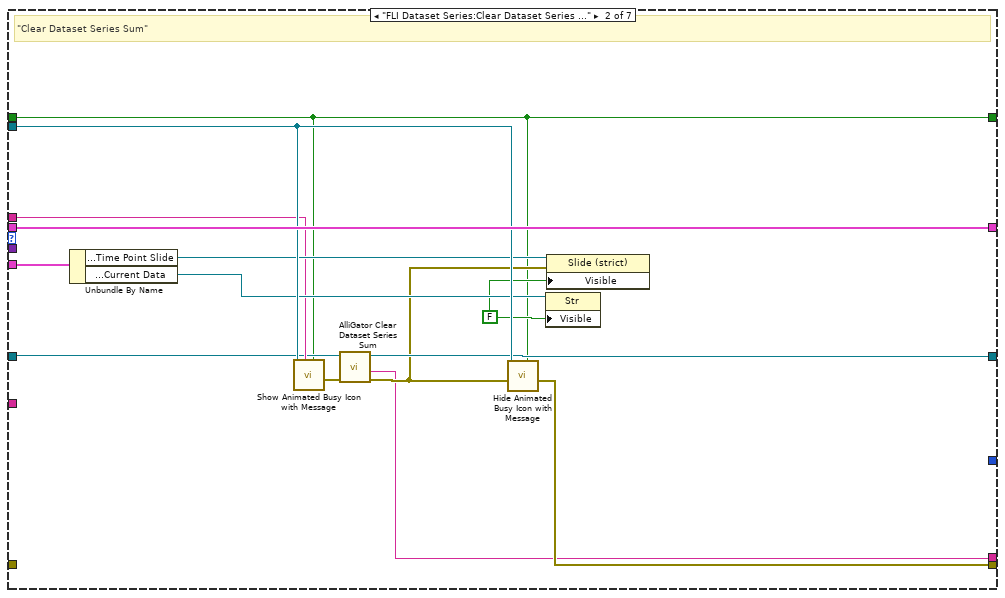
[diagram p3: hidden frame]
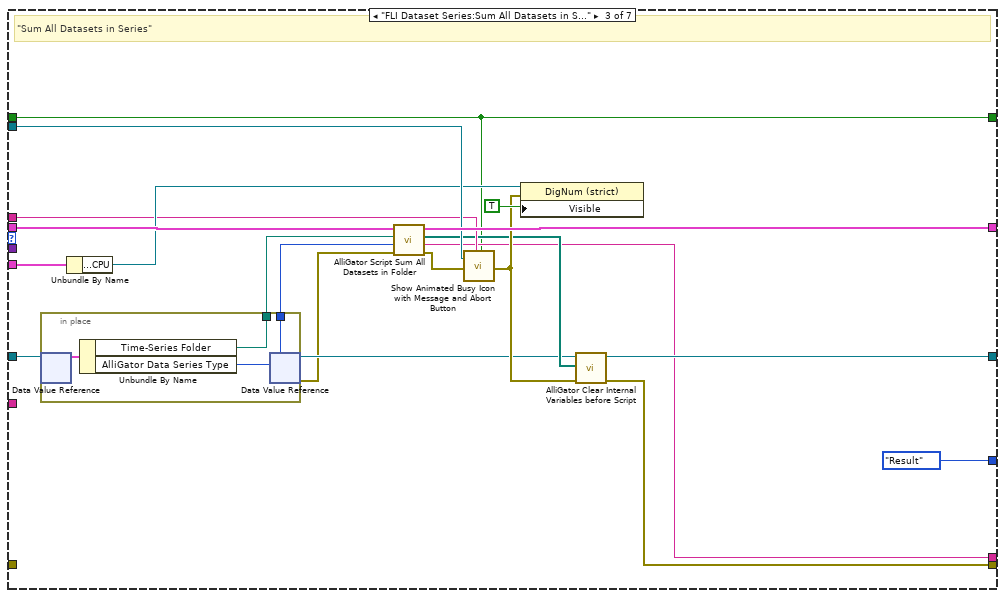
[diagram p4: hidden frame]
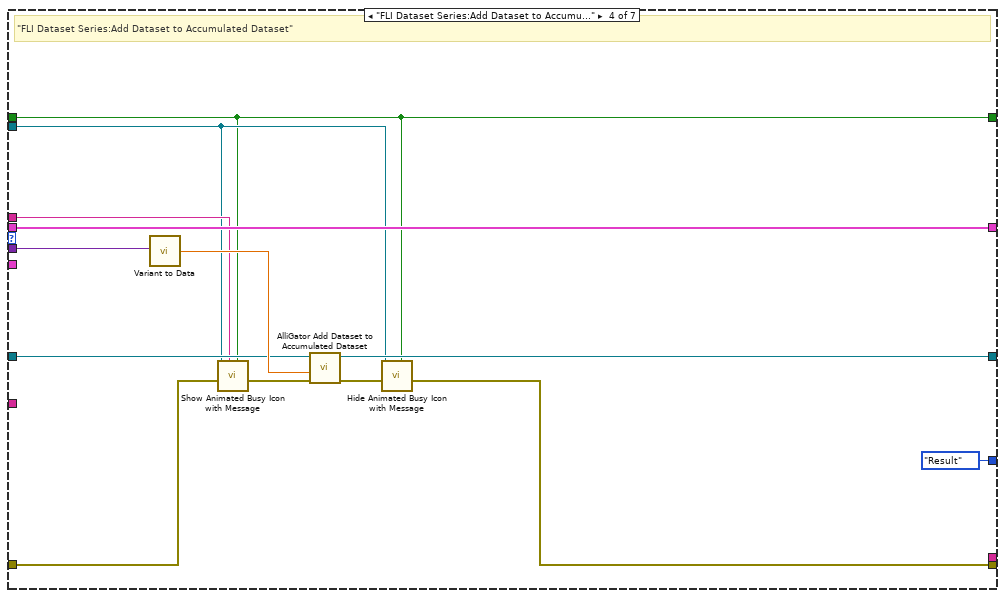
[diagram p5: hidden frame]
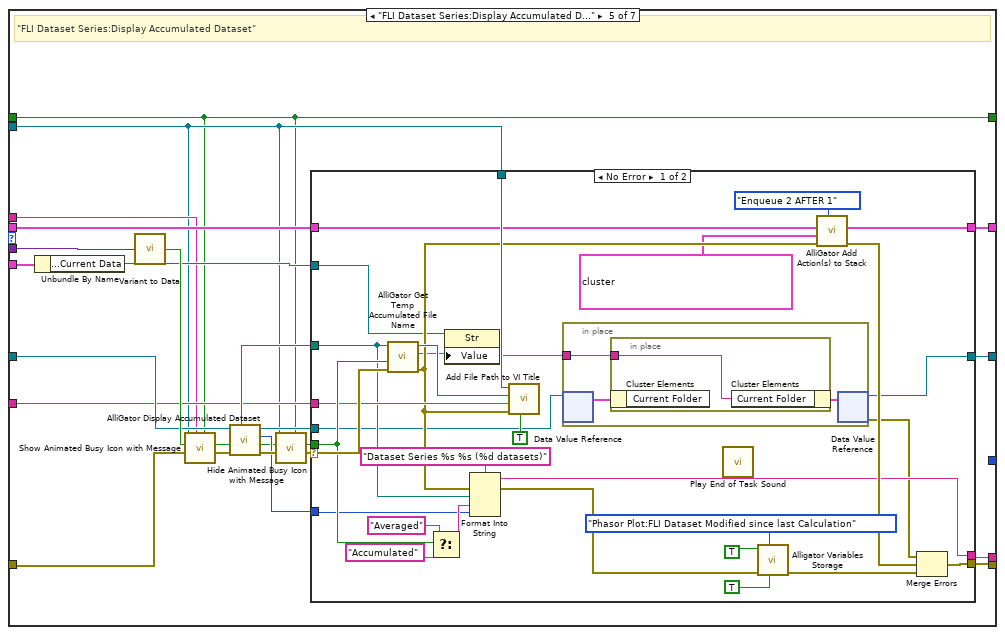
[diagram p6: hidden frame]
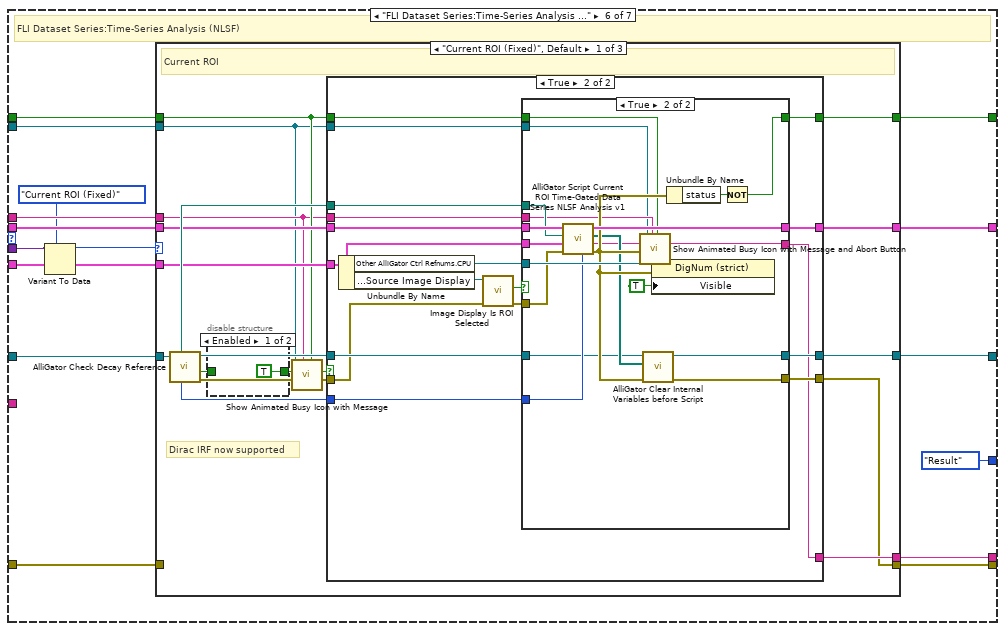
[diagram p8: hidden frame]
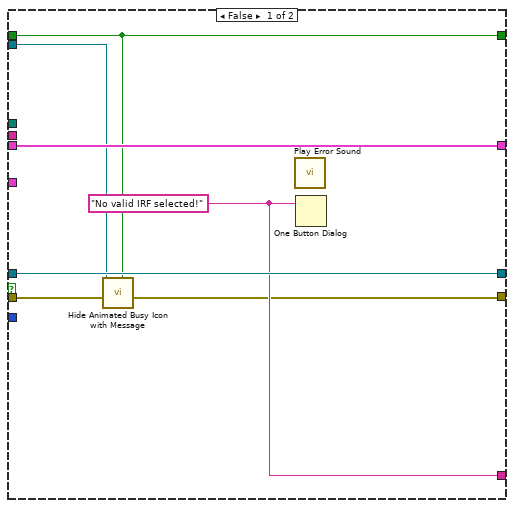
[diagram p10: hidden frame]
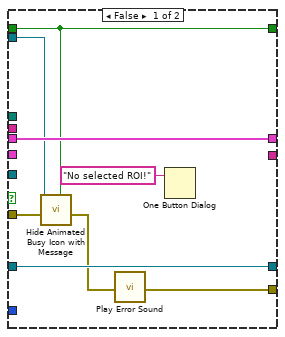
[diagram p11: hidden frame]
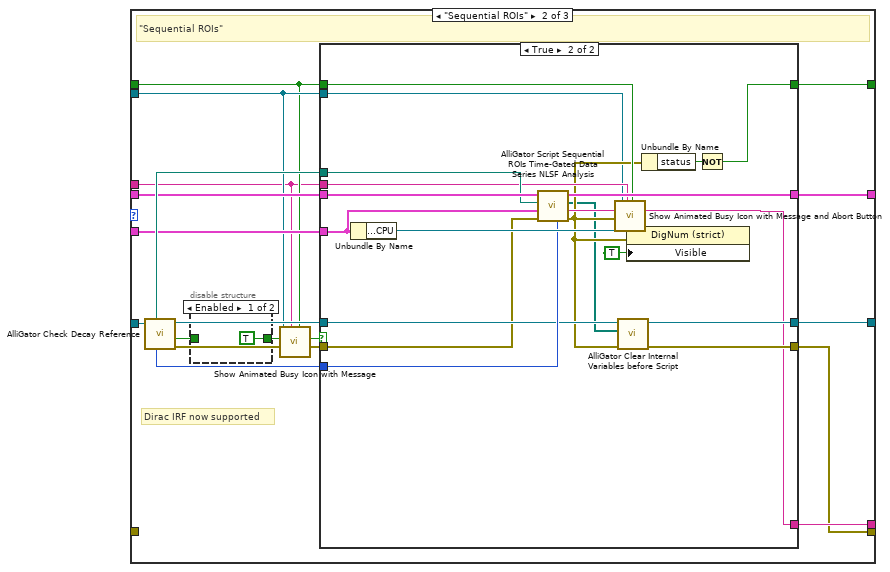
[diagram p12: hidden frame]
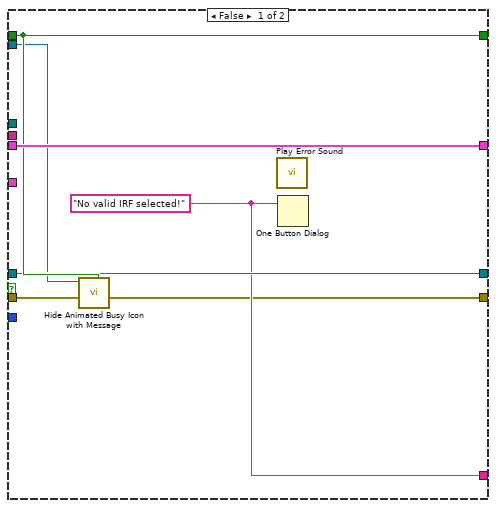
[diagram p14: hidden frame]
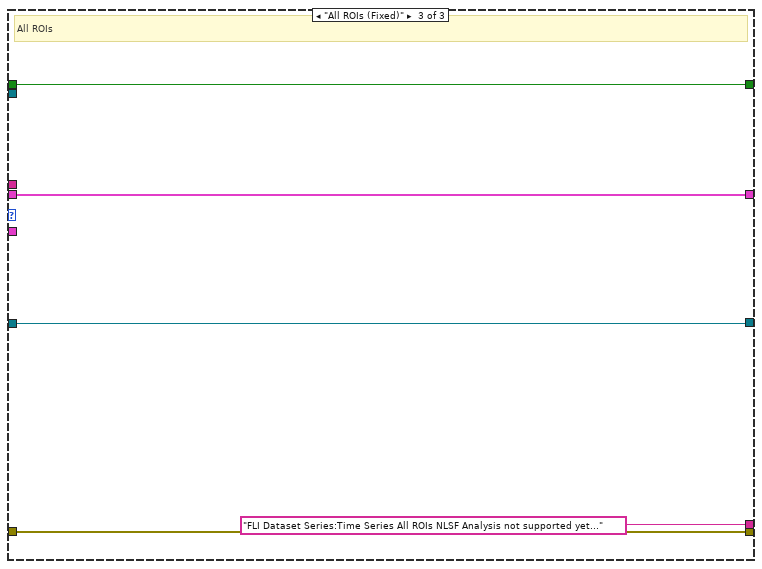
[diagram p15: hidden frame]
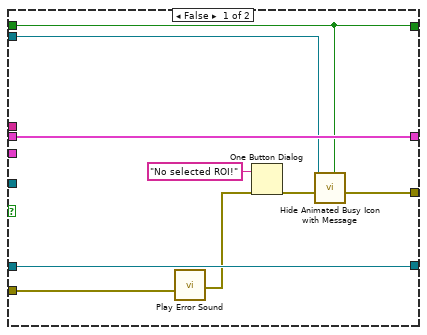
[diagram p16: hidden frame]
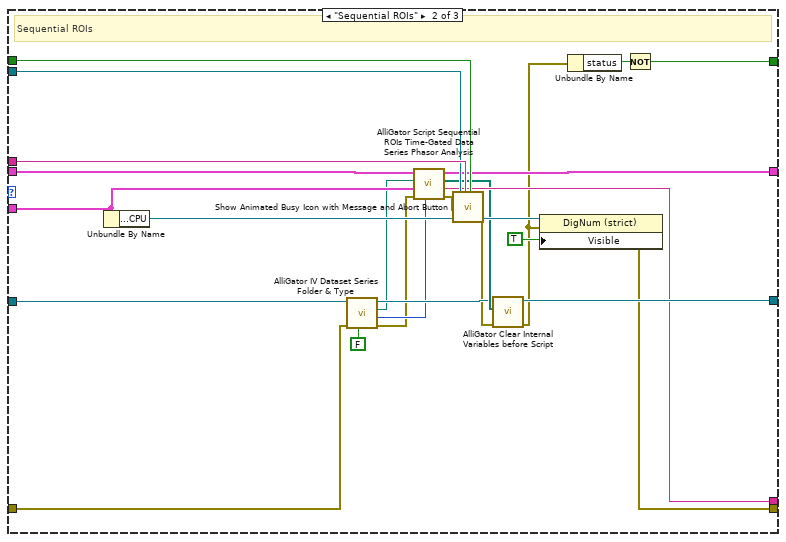
[diagram p17: hidden frame]
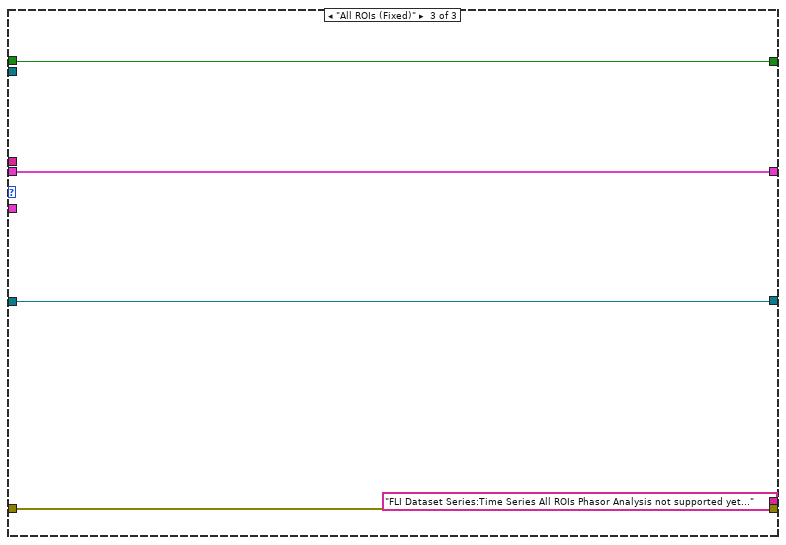
[diagram p18: hidden frame]
diagram:
  # "Author: Xavier Michalet\nCopyright 2025 REGENTS OF THE UNIVERSITY OF CALIFORNIA\n\nRedistribution and use in source and binary forms, with or without modification, are permitted provided that the following conditions are met:\n\n1. Redistributions of source code must retain the above copyright notice, this list of conditions and the following disclaimer.\n\n2. Redistributions in binary form must reproduce the above copyright notice, this list of conditions and the following disclaimer in the documentation and/or other materials provided with the distribution.\n\n3. Neither the name of the copyright holder nor the names of its contributors may be used to endorse or promote products derived from this software without specific prior written permission.\n\nTHIS SOFTWARE IS PROVIDED BY THE COPYRIGHT HOLDERS AND CONTRIBUTORS “AS IS” AND ANY EXPRESS OR IMPLIED WARRANTIES, INCLUDING, BUT NOT LIMITED TO, THE IMPLIED WARRANTIES OF MERCHANTABILITY AND FITNESS FOR A PARTICULAR PURPOSE ARE DISCLAIMED. IN NO EVENT SHALL THE COPYRIGHT HOLDER OR CONTRIBUTORS BE LIABLE FOR ANY DIRECT, INDIRECT, INCIDENTAL, SPECIAL, EXEMPLARY, OR CONSEQUENTIAL DAMAGES (INCLUDING, BUT NOT LIMITED TO, PROCUREMENT OF SUBSTITUTE GOODS OR SERVICES; LOSS OF USE, DATA, OR PROFITS; OR BUSINESS INTERRUPTION) HOWEVER CAUSED AND ON ANY THEORY OF LIABILITY, WHETHER IN CONTRACT, STRICT LIABILITY, OR TORT (INCLUDING NEGLIGENCE OR OTHERWISE) ARISING IN ANY WAY OUT OF THE USE OF THIS SOFTWARE, EVEN IF ADVISED OF THE POSSIBILITY OF SUCH DAMAGE."
  n1 = global read "AlliGator Globals.vi" "Alligator version"() -> (w8:string)
  n2 = call "AlliGator Event to String.vi"("AlliGator Q Event"="AlliGator Q Event in") -> ("String"=w9:string)  [unwired: 8 in]
  n3 = case shown="\"FLI Dataset Series:Time-Series Analysis (Phasor)\"" "AlliGator Q Event in" {
    tunnel: "Data" -> [_ _ _ w71 w86 w136 w275]
    tunnel: "AlliGator Q Elements" -> [w23 w37 w56 w73 w88 w146 w287]
    tunnel: [w23 w37 w57 w73 w87 w141 w278] -> w11
    tunnel: "VI in" -> [_ w36 w54 w63 w75 w147 w284]
    tunnel: [w22 w24 w39 w62 w74 w140 w277] -> w12
    tunnel: "Script in" -> [w22 w24 w39 w62 w74 w148 w283]
    tunnel: w9 -> [_ w30 w45 w64 w77 w139 w286]
    tunnel: "error in (no error)" -> [w21 _ _ w68 w80 w137 w276]
    tunnel: [w21 w35 w46 w65 w79 w143 w279] -> w1
    tunnel: "AlliGator Ctrl Refnums" -> [_ w34 w53 _ w85 w145 w285]
    tunnel: "AlliGator IV DVR in" -> [w20 w29 w42 w70 w84 w144 w282]
    tunnel: [w20 w27 w47 w67 w83 w142 w281] -> w19
    tunnel: [_ w25 w43 _ w81 w138 w280] -> w5
    tunnel: w8 -> [_ _ _ _ w82 _ _]
    tunnel: [_ _ Text_Format_List."Result" ("Text Format") Text_Format_List."Result" ("Text Format") _ Text_Format_List."Result" ("Text Format") Text_Format_List."Result" ("Text Format")] -> w3
    frame "---- FLI Dataset Series ----", Default {
    }
    frame "FLI Dataset Series:Clear Dataset Series Sum" {
      w31 = FALSE ("Visible")
      # "\"Clear Dataset Series Sum\""
      n4 = Unbundle By Name(w34) -> ("Dataset Control Refnums.Time Point Slide"=w33:refnum<vi>, "Dataset Control Refnums.Current Data"=w32:refnum<vi>)
      n5 = call "Show Animated Busy Icon with Message.vi"("Already active? (F)"=w24, "Message"=w30, "Target VI Refnum"=w36) -> ("Error Out"=w28:errorcluster)  [unwired: 8 in]
      n6 = call "AlliGator Clear Dataset Series Sum.vi"("error in (no error)"=w28, "Data Value Reference in"=w29) -> ("error out"=w26:errorcluster, "Message"=w25:string, "Data Value Reference out"=w27:refnum<data-value>)  [unwired: 7 in]
      n7 = call "Hide Animated Busy Icon with Message.vi"("Already active? (F)"=w24, "Error In"=w26, "Target VI reference"=w36) -> ("Error Out"=w35:errorcluster)  [unwired: 8 in]
      n8 = property class="Str"(reference=w32, "Visible"=w31) -> ()  [unwired: 1 in, 2 out]
      n9 = property class="Slide (strict)"(reference=w33, error in=w26, "Visible"=w31) -> ()  [unwired: 2 out]
    }
    frame "FLI Dataset Series:Sum All Datasets in Series" {
      # "\"Sum All Datasets in Series\""
      n10 = in-place {
        in-place-border: [w60] -> w49
        in-place-border: [w59] -> w48
        n11 = in-place-dvr #1(w42) -> (w58:T21)  [unwired: 1 out]
        n12 = Unbundle By Name(w58) -> ("Time-Series Folder"=w60:path, "AlliGator Data Series Type"=w59:T25)
        n13 = in-place-dvr #1() -> (w41:refnum<data-value>, w40:errorcluster)  [unwired: 1 in]
      }
      n14 = Unbundle By Name(w53) -> ("Other AlliGator Ctrl Refnums.CPU"=w50:refnum<vi>)
      n15 = call "AlliGator Script Sum All Datasets in Folder.vi"("Error In"=w40, "AlliGator Data Series Type"=w48, "Path"=w49, "Alligator Queue Elements in"=w56) -> ("Error Out"=w55:errorcluster, "Message"=w43:string, "[Time-Series Path]"=w44:path[], "Alligator Queue Elements out"=w57:T6[])  [unwired: 4 in]
      n16 = call "Show Animated Busy Icon with Message and Abort Button.vi"("Already active? (F)"=w39, "Message"=w45, "Target VI reference"=w54, "Error In"=w55) -> ("Error Out"=w51:errorcluster)  [unwired: 15 in]
      n17 = property class="DigNum (strict)"(reference=w50, error in=w51, "Visible"=TRUE) -> ()  [unwired: 2 out]
      n18 = call "AlliGator Clear Internal Variables before Script.vi"("Error In"=w51, "[Time-Series Path]"=w44, "AlliGator Internal Variables DVR in"=w41) -> ("Error Out"=w46:errorcluster, "AlliGator Internal Variables DVR out"=w47:refnum<data-value>)  [unwired: 7 in]
    }
    frame "FLI Dataset Series:Add Dataset to Accumulated Dataset" {
      # "\"FLI Dataset Series:Add Dataset to Accumulated Dataset\""
      n19 = call-poly "Variant to Data.vi"("Variant"=w71) -> ("Value"=w72:dbl)  [unwired: 8 in]
      n20 = call "Show Animated Busy Icon with Message.vi"("Already active? (F)"=w62, "Message"=w64, "Error In"=w68, "Target VI Refnum"=w63) -> ("Error Out"=w66:errorcluster)  [unwired: 7 in]
      n21 = call "AlliGator Add Dataset to Accumulated Dataset.vi"("error in (no error)"=w66, "Weight (1)"=w72, "AlliGator IV DVR in"=w70) -> ("error out"=w69:errorcluster, "AlliGator IV DVR out"=w67:refnum<data-value>)  [unwired: 7 in]
      n22 = call "Hide Animated Busy Icon with Message.vi"("Already active? (F)"=w62, "Error In"=w69, "Target VI reference"=w63) -> ("Error Out"=w65:errorcluster)  [unwired: 8 in]
    }
    frame "FLI Dataset Series:Display Accumulated Dataset" {
      # "\"FLI Dataset Series:Display Accumulated Dataset\""
      n23 = Unbundle By Name(w85) -> ("Dataset Control Refnums.Current Data"=w91:refnum<vi>)
      n24 = call-poly "Variant to Data.vi"("Variant"=w86) -> ("Value"=w92:bool)  [unwired: 8 in]
      n25 = call "Show Animated Busy Icon with Message.vi"("Already active? (F)"=w74, "Message"=w77, "Error In"=w80, "Target VI Refnum"=w75) -> ("Error Out"=w78:errorcluster)  [unwired: 7 in]
      n26 = call "AlliGator Display Accumulated Dataset.vi"("error in (no error)"=w78, "Sum (F) or Average (T)"=w92, "AlliGator IV DVR in"=w84) -> ("error out"=w94:errorcluster, "Averaged?"=w89:bool, "# Accumulated Datasets"=w90:i32, "AlliGator IV DVR out"=w95:refnum<data-value>, "Time-Series Folder"=w93:path)  [unwired: 4 in]
      n27 = call "Hide Animated Busy Icon with Message.vi"("Already active? (F)"=w74, "Error In"=w94, "Target VI reference"=w75) -> ("Error Out"=w76:errorcluster)  [unwired: 8 in]
      n28 = case shown="No Error" w76 {
        selector: w76 -> [w123 w132]
        tunnel: w75 -> [w125 _]
        tunnel: w93 -> [w115 _]
        tunnel: [w122 w132] -> w79
        tunnel: w89 -> [w118 _]
        tunnel: w82 -> [w116 _]
        tunnel: w90 -> [w113 _]
        tunnel: w88 -> [w112 w131]
        tunnel: [w111 w131] -> w87
        tunnel: w91 -> [w106 _]
        tunnel: w95 -> [w98 w130]
        tunnel: [w96 w130] -> w83
        tunnel: [w104 _] -> w81
        frame No Error {
          n29 = call "AlliGator Get Temp Accumulated File Name.vi"("error in (no error)"=w123, "Averaged?"=w118, "Time-Series Folder"=w115) -> ("error out"=w110:errorcluster, "filename without extension"=w105:string, "temporary file name"=w114:path)  [unwired: 6 in]
          n30 = Select(t="Averaged" ("string"), s=w118, f="Accumulated" ("string")) -> (s? t:f=w117:string)
          n31 = property class="Str"(reference=w106, "Value"=w105) -> ()  [unwired: 1 in, 2 out]
          n32 = Format Into String(format string="Dataset Series %s %s (%d datasets)" ("initial string"), error in=w110, w115, w117, w113) -> (resulting string=w104:string, error out=w103:errorcluster)  [unwired: 1 in]
          n33 = call "Add File Path to VI Title.vi"("Add Asterisk?"=TRUE, "Error In"=w110, "VI Title"=w116, "File Path"=w114, "VI Refnum"=w125) -> ()  [unwired: 6 in, 1 out]
          n34 = in-place {
            in-place-border: w105 -> [w128]
            n35 = in-place-dvr #2(w98) -> (w127:T21)  [unwired: 1 out]
            n36 = in-place {
              in-place-border: w128 -> [w129]
              n37 = in-place-cluster #3(w127) -> ()  [unwired: 1 out]
              n38 = in-place-cluster #3("Current Folder"=w129) -> (w126:T21)
            }
            n39 = in-place-dvr #2(w126) -> (w96:refnum<data-value>, w97:errorcluster)
          }
          n40 = call "Play End of Task Sound.vi"() -> ()  [unwired: 27 in, 1 out]
          n41 = call "Alligator Variables Storage.vi"("Get(F)/Set"=TRUE, "AlliGator Variable"=AlliGator_Variables_List."Phasor Plot:FLI Dataset Modified since last Calculation" ("Alligator Variable"), "Error In"=w103, "Data in"=TRUE) -> ("Error Out"=w102:errorcluster)  [unwired: 5 in, 2 out]
          n42 = call-poly "AlliGator Add Action(s) to Stack.vi"("Elements Order in Action Stack (Default: 2 BEFORE 1)"=Alligator_Elements_Order_in_Action_Stack."Enqueue 2 AFTER 1", "Error In"=w110, "Alligator Queue Element 2"=T6[] [{"AlliGator Q Event"=enum."Image:Image Histogram", "Data"=variant}, {"AlliGator Q Event"=enum."Image:Image Contrast", "Data"=variant}] ("Alligator Atomic Action"), "Alligator Queue Element 1"=w112) -> ("Error Out"=w109:errorcluster, "Alligator Queue Element 1 (+ 2)"=w111:T6[])  [unwired: 6 in]
          n43 = Merge Errors(w97, w109, w102) -> (w122:errorcluster)
        }
        frame Error {
        }
      }
    }
    frame "FLI Dataset Series:Time-Series Analysis (NLSF)" {
      # "FLI Dataset Series:Time-Series Analysis (NLSF)"
      n44 = Variant To Data(type=AlliGator_Series_Analysis_Type."Current ROI (Fixed)" ("Series Analysis Type"), Variant=w136) -> (data=w134:T20)  [unwired: 1 in, 1 out]
      n45 = case shown="\"Current ROI (Fixed)\", Default" w134 {
        tunnel: w148 -> [w152 w224 w271]
        tunnel: w147 -> [w150 w225 _]
        tunnel: w146 -> [w162 w234 w270]
        tunnel: w145 -> [w161 w233 _]
        tunnel: w144 -> [w160 w232 w269]
        tunnel: [w149 w221 w268] -> w143
        tunnel: [w159 w231 w269] -> w142
        tunnel: [w158 w230 w270] -> w141
        tunnel: [w157 w222 w271] -> w140
        tunnel: w139 -> [w151 w223 _]
        tunnel: [w156 w229 "FLI Dataset Series:Time Series All ROIs NLSF Analysis not supported yet..." ("Message")] -> w138
        tunnel: w137 -> [_ _ w268]
        frame "Current ROI (Fixed)", Default {
          # "Dirac IRF now supported"
          # "Current ROI"
          n46 = call "AlliGator Check Decay Reference.vi"("AlliGator Internal Variables DVR"=w160) -> ("Error Out"=w163:errorcluster, "Valid Reference?"=w155:bool, "AlliGator Internal Variables DVR"=w164:refnum<data-value>, "AlliGator Data Series Type"=w165:T25, "Time-Series Folder"=w166:path)  [unwired: 3 in, 3 out]
          n47 = disable-structure shown="Enabled" {
            disable-tunnel: w155 -> [_ w168]
            disable-tunnel: [TRUE ("Valid Reference?") w168] -> w154
            frame Enabled {
            }
            frame Disabled {
            }
          }
          n48 = call "Show Animated Busy Icon with Message.vi"("Already active? (F)"=w152, "Message"=w151, "Error In"=w163, "Target VI Refnum"=w150) -> ("Error Out"=w153:errorcluster)  [unwired: 7 in]
          n49 = case shown="True" w154 {
            tunnel: [w175 w193] -> w158
            tunnel: [w171 w187] -> w149
            tunnel: w162 -> [w175 w192]
            tunnel: w152 -> [w169 w182]
            tunnel: [w169 w191] -> w157
            tunnel: w161 -> [_ w176]
            tunnel: w153 -> [w172 w179]
            tunnel: w150 -> [w170 w190]
            tunnel: [w174 w188] -> w159
            tunnel: w166 -> [_ w186]
            tunnel: w165 -> [_ w185]
            tunnel: w164 -> [w174 w184]
            tunnel: w151 -> [_ w183]
            tunnel: [w173 w181] -> w156
            frame False {
              w173 = "No valid IRF selected!" ("Script Message")
              n50 = call "Hide Animated Busy Icon with Message.vi"("Already active? (F)"=w169, "Error In"=w172, "Target VI reference"=w170) -> ("Error Out"=w171:errorcluster)  [unwired: 8 in]
              n51 = call "Play Error Sound.vi"() -> ()  [unwired: 27 in, 1 out]
              n52 = One Button Dialog(message=w173) -> ()  [unwired: 1 in, 1 out]
            }
            frame True {
              n53 = Unbundle By Name(w176) -> ("Other AlliGator Ctrl Refnums.CPU"=w189:refnum<vi>, "Registered Events Ctrl Refnums.Source Image Display"=w180:refnum<vi>)
              n54 = call "Image Display Is ROI Selected.vi"("Error In"=w179, "Image Control Refnum"=w180) -> ("Error Out"=w178:errorcluster, "Is ROI Selected?"=w177:bool)  [unwired: 7 in, 1 out]
              n55 = case shown="True" w177 {
                tunnel: [w201 w220] -> w193
                tunnel: w192 -> [w201 w219]
                tunnel: [w194 w217] -> w191
                tunnel: w190 -> [w195 w202]
                tunnel: w189 -> [_ w216]
                tunnel: [w200 w212] -> w188
                tunnel: [w198 w211] -> w187
                tunnel: w186 -> [_ w210]
                tunnel: w185 -> [_ w209]
                tunnel: w184 -> [w200 w208]
                tunnel: w183 -> [_ w207]
                tunnel: w182 -> [w194 w206]
                tunnel: [_ w205] -> w181
                tunnel: w178 -> [w199 w204]
                tunnel: w176 -> [_ w203]
                frame False {
                  n56 = call "Hide Animated Busy Icon with Message.vi"("Already active? (F)"=w194, "Error In"=w199, "Target VI reference"=w195) -> ("Error Out"=w196:errorcluster)  [unwired: 8 in]
                  n57 = call "Play Error Sound.vi"("Error In"=w196) -> ("Error Out"=w198:errorcluster)  [unwired: 26 in]
                  n58 = One Button Dialog(message="No selected ROI!") -> ()  [unwired: 1 in, 1 out]
                }
                frame True {
                  n59 = call "AlliGator Script Current ROI Time-Gated Data Series NLSF Analysis v1.vi"("AlliGator Data Series Type"=w209, "Error In"=w204, "AlliGator Ctrl Refnums"=w203, "Path"=w210, "Alligator Queue Elements in"=w219) -> ("Error Out"=w215:errorcluster, "Message"=w205:string, "Time-Series Paths"=w213:path[], "Alligator Queue Elements out"=w220:T6[])  [unwired: 3 in]
                  n60 = call "Show Animated Busy Icon with Message and Abort Button.vi"("Already active? (F)"=w206, "Message"=w207, "Target VI reference"=w202, "Error In"=w215) -> ()  [unwired: 15 in, 1 out]
                  n61 = call "AlliGator Clear Internal Variables before Script.vi"("Error In"=w215, "[Time-Series Path]"=w213, "AlliGator Internal Variables DVR in"=w208) -> ("Error Out"=w211:errorcluster, "AlliGator Internal Variables DVR out"=w212:refnum<data-value>)  [unwired: 7 in]
                  n62 = property class="DigNum (strict)"(reference=w216, error in=w215, "Visible"=TRUE) -> ()  [unwired: 2 out]
                  n63 = Unbundle By Name(w215) -> ("status"=w218:bool)
                  n64 = Not(x=w218) -> (.not. x?=w217:bool)
                }
              }
            }
          }
        }
        frame "Sequential ROIs" {
          # "Dirac IRF now supported"
          # "\"Sequential ROIs\""
          n65 = call "AlliGator Check Decay Reference.vi"("AlliGator Internal Variables DVR"=w232) -> ("Error Out"=w235:errorcluster, "Valid Reference?"=w228:bool, "AlliGator Internal Variables DVR"=w236:refnum<data-value>, "AlliGator Data Series Type"=w237:T25, "Time-Series Folder"=w238:path)  [unwired: 3 in, 3 out]
          n66 = disable-structure shown="Enabled" {
            disable-tunnel: w228 -> [_ w240]
            disable-tunnel: [TRUE ("Valid Reference?") w240] -> w227
            frame Enabled {
            }
            frame Disabled {
            }
          }
          n67 = call "Show Animated Busy Icon with Message.vi"("Already active? (F)"=w224, "Message"=w223, "Error In"=w235, "Target VI Refnum"=w225) -> ("Error Out"=w226:errorcluster)  [unwired: 7 in]
          n68 = case shown="True" w227 {
            tunnel: [w247 w266] -> w230
            tunnel: [w241 w261] -> w221
            tunnel: w234 -> [w247 w265]
            tunnel: w224 -> [w246 w256]
            tunnel: [w246 w264] -> w222
            tunnel: w233 -> [_ w254]
            tunnel: w226 -> [w243 w253]
            tunnel: w225 -> [w242 w248]
            tunnel: [w245 w262] -> w231
            tunnel: w238 -> [_ w260]
            tunnel: w237 -> [_ w259]
            tunnel: w236 -> [w245 w258]
            tunnel: w223 -> [_ w257]
            tunnel: [w244 w255] -> w229
            frame False {
              w244 = "No valid IRF selected!" ("Script Message")
              n69 = call "Hide Animated Busy Icon with Message.vi"("Already active? (F)"=w246, "Error In"=w243, "Target VI reference"=w242) -> ("Error Out"=w241:errorcluster)  [unwired: 8 in]
              n70 = call "Play Error Sound.vi"() -> ()  [unwired: 27 in, 1 out]
              n71 = One Button Dialog(message=w244) -> ()  [unwired: 1 in, 1 out]
            }
            frame True {
              n72 = Unbundle By Name(w254) -> ("Other AlliGator Ctrl Refnums.CPU"=w263:refnum<vi>)
              n73 = call "AlliGator Script Sequential ROIs Time-Gated Data Series NLSF Analysis.vi"("AlliGator Data Series Type"=w259, "Error In"=w253, "AlliGator Ctrl Refnums"=w254, "Path"=w260, "Alligator Queue Elements in"=w265) -> ("Error Out"=w251:errorcluster, "Message"=w255:string, "Time-Series Paths"=w249:path[], "Alligator Queue Elements out"=w266:T6[])  [unwired: 3 in]
              n74 = call "Show Animated Busy Icon with Message and Abort Button.vi"("Already active? (F)"=w256, "Message"=w257, "Target VI reference"=w248, "Error In"=w251) -> ()  [unwired: 15 in, 1 out]
              n75 = call "AlliGator Clear Internal Variables before Script.vi"("Error In"=w251, "[Time-Series Path]"=w249, "AlliGator Internal Variables DVR in"=w258) -> ("Error Out"=w261:errorcluster, "AlliGator Internal Variables DVR out"=w262:refnum<data-value>)  [unwired: 7 in]
              n76 = property class="DigNum (strict)"(reference=w263, error in=w251, "Visible"=TRUE) -> ()  [unwired: 2 out]
              n77 = Unbundle By Name(w251) -> ("status"=w252:bool)
              n78 = Not(x=w252) -> (.not. x?=w264:bool)
            }
          }
        }
        frame "All ROIs (Fixed)" {
          # "All ROIs"
        }
      }
    }
    frame "FLI Dataset Series:Time-Series Analysis (Phasor)" {
      # "\"FLI Dataset Series:Time Series Analysis (Phasor)\""
      n79 = Variant To Data(type=AlliGator_Series_Analysis_Type."Current ROI (Fixed)" ("Series Analysis Type"), Variant=w275) -> (data=w273:T20)  [unwired: 1 in, 1 out]
      n80 = case shown="\"Current ROI (Fixed)\", Default" w273 {
        tunnel: w287 -> [w303 w359 w364]
        tunnel: w286 -> [w288 w358 _]
        tunnel: w285 -> [w292 w348 _]
        tunnel: w284 -> [w290 w357 _]
        tunnel: w283 -> [w289 w356 w365]
        tunnel: w282 -> [w302 w355 w363]
        tunnel: [w301 w354 w363] -> w281
        tunnel: [w300 w353 "FLI Dataset Series:Time Series All ROIs Phasor Analysis not supported yet..." ("Message")] -> w280
        tunnel: [w299 w352 w362] -> w279
        tunnel: [w298 w351 w364] -> w278
        tunnel: [w297 w350 w365] -> w277
        tunnel: w276 -> [w295 w349 w362]
        frame "Current ROI (Fixed)", Default {
          # "Current ROI"
          n81 = Unbundle By Name(w292) -> ("Other AlliGator Ctrl Refnums.CPU"=w304:refnum<vi>, "Registered Events Ctrl Refnums.Source Image Display"=w296:refnum<vi>)
          n82 = call "Image Display Is ROI Selected.vi"("Error In"=w295, "Image Control Refnum"=w296) -> ("Error Out"=w294:errorcluster, "Is ROI Selected?"=w293:bool)  [unwired: 7 in, 1 out]
          n83 = call "Show Animated Busy Icon with Message.vi"("Already active? (F)"=w289, "Message"=w288, "Error In"=w294, "Target VI Refnum"=w290) -> ("Error Out"=w291:errorcluster)  [unwired: 7 in]
          n84 = case shown="True" w293 {
            tunnel: w304 -> [_ w334]
            tunnel: w303 -> [w312 w326]
            tunnel: w288 -> [_ w325]
            tunnel: w290 -> [w306 w324]
            tunnel: w289 -> [w305 w323]
            tunnel: w302 -> [w311 w322]
            tunnel: [w311 w321] -> w301
            tunnel: [_ w315] -> w300
            tunnel: [w307 w320] -> w299
            tunnel: [w312 w319] -> w298
            tunnel: [w305 w317] -> w297
            tunnel: w291 -> [w309 w313]
            tunnel: w292 -> [_ w314]
            frame False {
              n85 = call "Play Error Sound.vi"("Error In"=w309) -> ("Error Out"=w308:errorcluster)  [unwired: 26 in]
              n86 = One Button Dialog(message="No selected ROI!") -> ()  [unwired: 1 in, 1 out]
              n87 = call "Hide Animated Busy Icon with Message.vi"("Already active? (F)"=w305, "Error In"=w308, "Target VI reference"=w306) -> ("Error Out"=w307:errorcluster)  [unwired: 8 in]
            }
            frame True {
              n88 = call "AlliGator IV Dataset Series Folder & Type.vi"("Get (F)/ Set (T)"=FALSE, "error in (no error)"=w313, "AlliGator IV DVR in"=w322) -> ("error out"=w328:errorcluster, "AlliGator Data Series Type"=w329:T25, "Time-Series Folder"=w330:path, "AlliGator IV DVR out"=w331:refnum<data-value>)  [unwired: 4 in, 1 out]
              n89 = call "AlliGator Script Current ROI Time-Gated Data Series Phasor Analysis v2.vi"("AlliGator Data Series Type"=w329, "Error In"=w328, "AlliGator Ctrl Refnums"=w314, "Path"=w330, "Alligator Queue Elements in"=w326) -> ("Error Out"=w335:errorcluster, "Message"=w315:string, "Time-Series Paths"=w332:path[], "Alligator Queue Elements out"=w319:T6[])  [unwired: 3 in]
              n90 = call "Show Animated Busy Icon with Message and Abort Button.vi"("Already active? (F)"=w323, "Message"=w325, "Target VI reference"=w324, "Error In"=w335) -> ("Error Out"=w318:errorcluster)  [unwired: 15 in]
              n91 = call "AlliGator Clear Internal Variables before Script.vi"("Error In"=w318, "[Time-Series Path]"=w332, "AlliGator Internal Variables DVR in"=w331) -> ("Error Out"=w316:errorcluster, "AlliGator Internal Variables DVR out"=w321:refnum<data-value>)  [unwired: 7 in]
              n92 = property class="DigNum (strict)"(reference=w334, error in=w316, "Visible"=TRUE) -> (error out=w320:errorcluster)  [unwired: 1 out]
              n93 = Unbundle By Name(w316) -> ("status"=w336:bool)
              n94 = Not(x=w336) -> (.not. x?=w317:bool)
            }
          }
        }
        frame "Sequential ROIs" {
          # "Sequential ROIs"
          n95 = Unbundle By Name(w348) -> ("Other AlliGator Ctrl Refnums.CPU"=w360:refnum<vi>)
          n96 = call "AlliGator IV Dataset Series Folder & Type.vi"("Get (F)/ Set (T)"=FALSE, "error in (no error)"=w349, "AlliGator IV DVR in"=w355) -> ("error out"=w340:errorcluster, "AlliGator Data Series Type"=w341:T25, "Time-Series Folder"=w342:path, "AlliGator IV DVR out"=w343:refnum<data-value>)  [unwired: 4 in, 1 out]
          n97 = call "AlliGator Script Sequential ROIs Time-Gated Data Series Phasor Analysis.vi"("AlliGator Data Series Type"=w341, "Error In"=w340, "AlliGator Ctrl Refnums"=w348, "Path"=w342, "Alligator Queue Elements in"=w359) -> ("Error Out"=w346:errorcluster, "Message"=w353:string, "Time-Series Paths"=w344:path[], "Alligator Queue Elements out"=w351:T6[])  [unwired: 3 in]
          n98 = call "Show Animated Busy Icon with Message and Abort Button.vi"("Already active? (F)"=w356, "Message"=w358, "Target VI reference"=w357, "Error In"=w346) -> ("Error Out"=w338:errorcluster)  [unwired: 15 in]
          n99 = call "AlliGator Clear Internal Variables before Script.vi"("Error In"=w338, "[Time-Series Path]"=w344, "AlliGator Internal Variables DVR in"=w343) -> ("Error Out"=w337:errorcluster, "AlliGator Internal Variables DVR out"=w354:refnum<data-value>)  [unwired: 7 in]
          n100 = property class="DigNum (strict)"(reference=w360, error in=w337, "Visible"=TRUE) -> (error out=w352:errorcluster)  [unwired: 1 out]
          n101 = Unbundle By Name(w337) -> ("status"=w347:bool)
          n102 = Not(x=w347) -> (.not. x?=w350:bool)
        }
        frame "All ROIs (Fixed)" {
        }
      }
    }
  }
  "AlliGator IV DVR out" <- w19
  "error out" <- w1
  "Script out" <- w12
  "Alligator Queue Elements" <- w11
  n103 = call "Get Current Message Text Format.vi"("Text Format"=w3) -> ("Error Out"=w2:errorcluster, "Message Formatting"=w4:T2)  [unwired: 8 in]
  n104 = call "AlliGator Package Notebook Messages.vi"("Error In"=w2, "Message Formatting"=w4, "Message"=w5, "AlliGator Q Event in"="AlliGator Q Event in") -> ("[Notebook Message]"=→"[Notebook Message]":T1[])  [unwired: 6 in, 1 out]
